vi "Interpolate_Calib_Coeff.vi"(5 "Analysis Info cluster":T1={"Colour"=0, "Inst type"=enum."Pitot-static tube", "Inst name"="Manometer voltage", "Symbol"="U", "Code name"="", "Extra Info"="U", "Inst Array"=enum."PWA", "Extra Titles"=[], "Extra Values"=[], "U"=0.0, "u^2"=0.0, "u^3"=0.0, "u^4"=0.0, "Skew_u"=0.0, "Kurt_u"=0.0, "Sd Error in Mean"=0.0, "% u'/U"=0.0, "X"=0.0, "Y"=0.0, "Z"=0.0, "Timescale integral to 25%"=0.0, "Sd Error in Variance"=0.0, "Calib File"=path "", "Calib Constants"=[], "Output Position"=FALSE, "Full Stats"=FALSE, "Av Sampling Rate"=0.0, "Av No of Samples"=0.0, "Total Meas Time (s)"=0.0, "ADAM Ch Name"="", "Max value"=0.0, "Min value"=0.0} {"Sd Error in Variance" format="%.2f"; "Skew_u" format="%.2f"; "% u'/U" format="%.2f"; "Sd Error in Mean" format="%.2f"; "Kurt_u" format="%.2f"; "u^4" format="%.2f"; "u^3" format="%.2f"; "U" format="%.2f"; "u^2" format="%.2f"}, 7 "Take New Data?":bool) -> (0 "Calib Coeff":dbl[](array[numeric]), 1 "Calib Type Name":string, 2 "Calib file string":string, 3 "Read file":bool, 4 "Analysis Info cluster  Out":T1={"Colour"=0, "Inst type"=enum."Pitot-static tube", "Inst name"="Manometer voltage", "Symbol"="U", "Code name"="", "Extra Info"="U", "Inst Array"=enum."PWA", "Extra Titles"=[], "Extra Values"=[], "U"=0.0, "u^2"=0.0, "u^3"=0.0, "u^4"=0.0, "Skew_u"=0.0, "Kurt_u"=0.0, "Sd Error in Mean"=0.0, "% u'/U"=0.0, "X"=0.0, "Y"=0.0, "Z"=0.0, "Timescale integral to 25%"=0.0, "Sd Error in Variance"=0.0, "Calib File"=path "", "Calib Constants"=[], "Output Position"=FALSE, "Full Stats"=FALSE, "Av Sampling Rate"=0.0, "Av No of Samples"=0.0, "Total Meas Time (s)"=0.0, "ADAM Ch Name"="", "Max value"=0.0, "Min value"=0.0} {"Sd Error in Variance" format="%.2f"; "Skew_u" format="%.2f"; "% u'/U" format="%.2f"; "Sd Error in Mean" format="%.2f"; "Kurt_u" format="%.2f"; "u^4" format="%.2f"; "u^3" format="%.2f"; "U" format="%.2f"; "u^2" format="%.2f"})   [LabVIEW 2015]
uses:
  Controls/Analysis_info_cluster.ctl
  Controls/Inst_type.ctl
  Controls/Instrument_Array.ctl
  XW calib map/Map method.ctl
  Globals/Meas_global.vi
  XW calib map/XW_Map_Global.vi
  Globals/Plug_in_data_global.vi
  Globals/Dynamic_call_global.ph.vi
  <vilib>/Analysis/NI_AALPro.lvlib
panel:
  out "Volts":dbl
  out "Time":dbl format="%#.0f"
  out "Earlier raw data file":string
  in  "TAKE NEW DATA XW Map method":T4=enum."Const. Psi_eff (std.)"
  in  "Domain padding factor":dbl=1.01
  in  "cap indicial sum to n":bool=TRUE
  in  "surface order (n)":i32=5
  in  "Apply calibration corrections":bool=TRUE
  in  "POST PROC. XW Map method":T4=enum."Psi_eff, k = f(Umagn.)"
  in  "variable n":bool=TRUE
  in  "wire diameter (mu.m)":dbl=5.0
  out "Header info":string[][](array[string])
  # "For polysurface method only:"
  # "For trimesh method only"
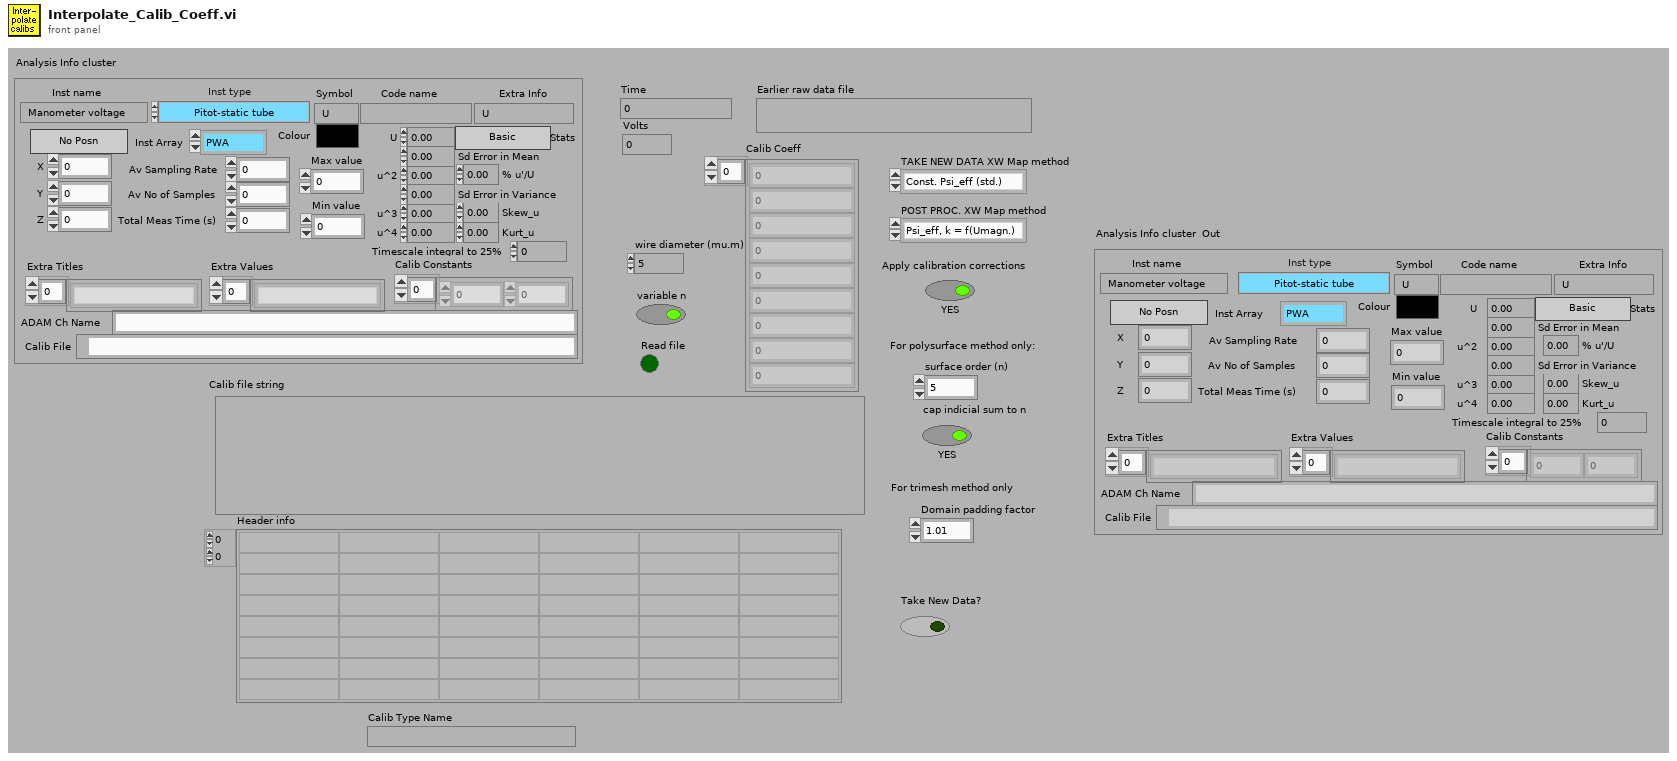
[diagram p1: front panel]
types:
  T1 = typedef "Analysis_info_cluster.ctl" = cluster{"Colour":u32, "Inst type":T2, "Inst name":string, "Symbol":string, "Code name":string, "Extra Info":string, "Inst Array":T3, "Extra Titles":string[], "Extra Values":string[], "U":dbl, "u^2":dbl, "u^3":dbl, "u^4":dbl, "Skew_u":dbl, "Kurt_u":dbl, "Sd Error in Mean":dbl, "% u'/U":dbl, "X":dbl, "Y":dbl, "Z":dbl, "Timescale integral to 25%":dbl, "Sd Error in Variance":dbl, "Calib File":path, "Calib Constants":dbl[], "Output Position":bool, "Full Stats":bool, "Av Sampling Rate":dbl, "Av No of Samples":dbl, "Total Meas Time (s)":dbl, "ADAM Ch Name":string, "Max value":dbl, "Min value":dbl}
  T2 = typedef "Inst_type.ctl" = enum16{"Propeller anemometer", "Raw voltage", "Pressure Transducer", "Pitot-static tube", "Preston tube", "Hot wire", "Cross wire 1", "Cross wire 2", "Generic Linear", "Generic Polynomial", "Generic BackPoly", "Fast FID", "Thermocouple", "Cold wire", "Pulsed Wire", "LDA Vel", "LDA Tran time", "LDA Arr time", "Microphone"}
  T3 = typedef "Instrument_Array.ctl" = enum16{"PWA", "LDA", "Analogue"}
  T4 = typedef "Map method.ctl" = enum16{"Triangle mesh", "Polynomial surface", "Const. Psi_eff (std.)", "Psi_eff = f(Umagn.)", "Psi_eff, k = f(Umagn.)"}
  T5 = cluster{"1st Calib time":dbl, "2nd Calib time":dbl, "Meas start time":dbl, "Meas end time":dbl, "Fraction":dbl}
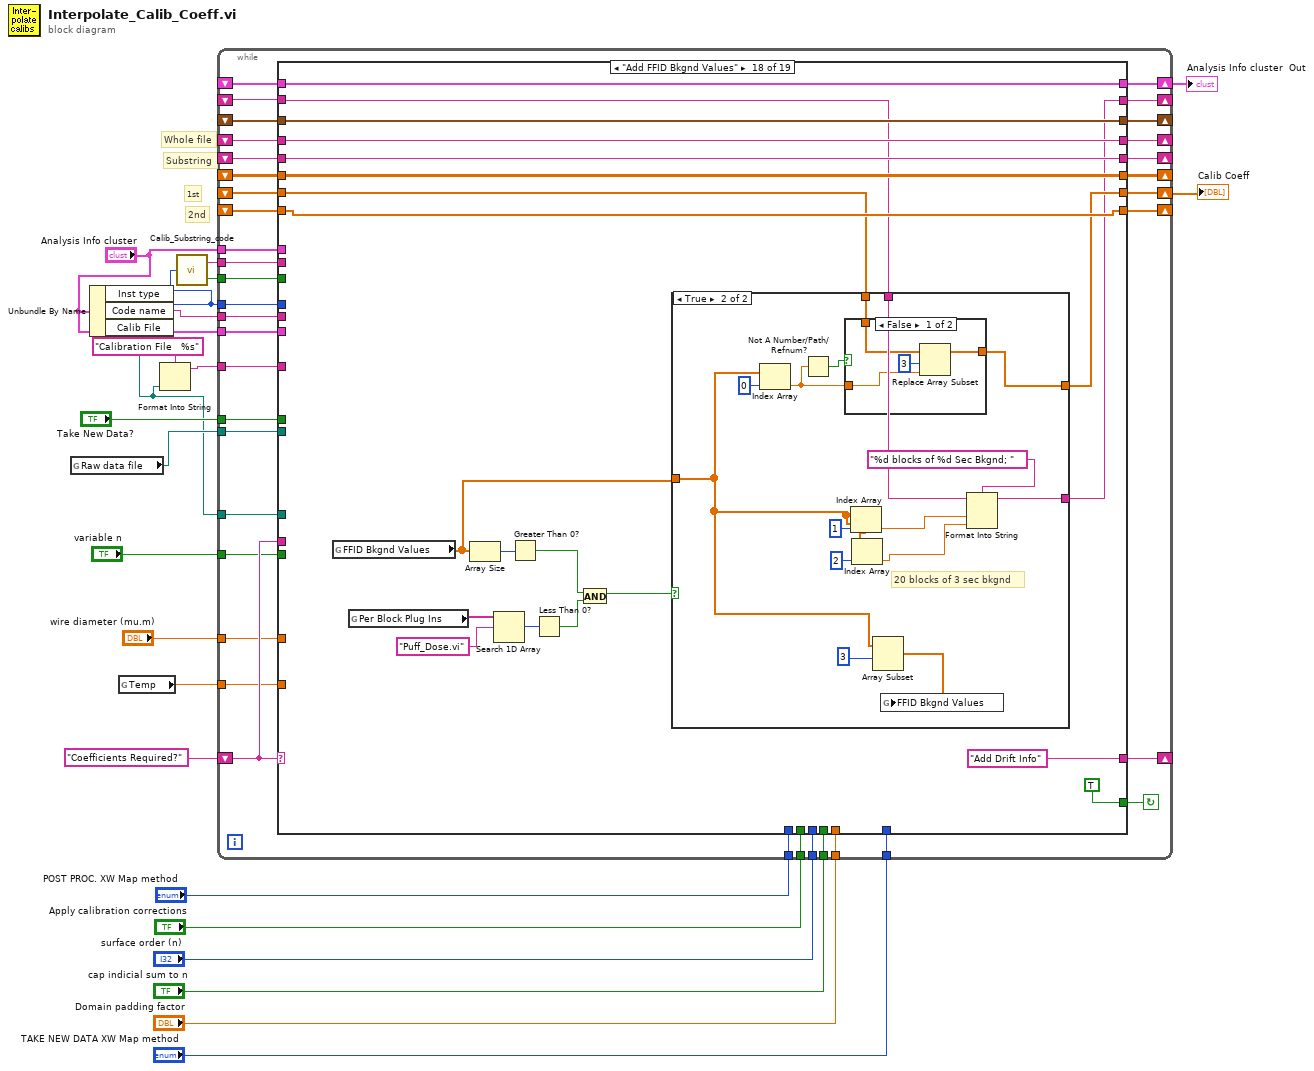
[diagram p0: block diagram]
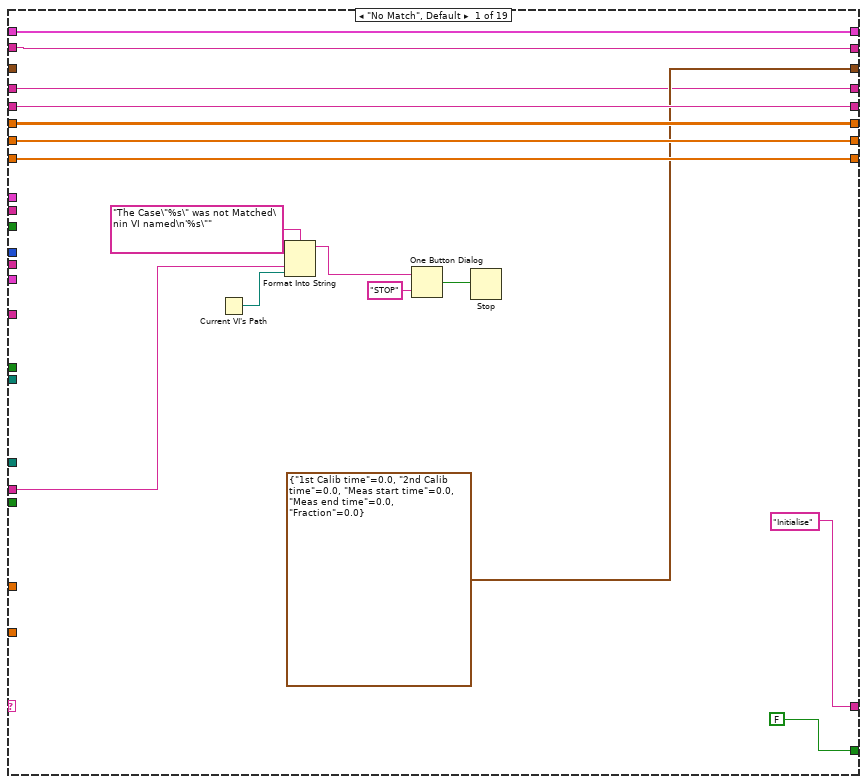
[diagram p2: hidden frame]
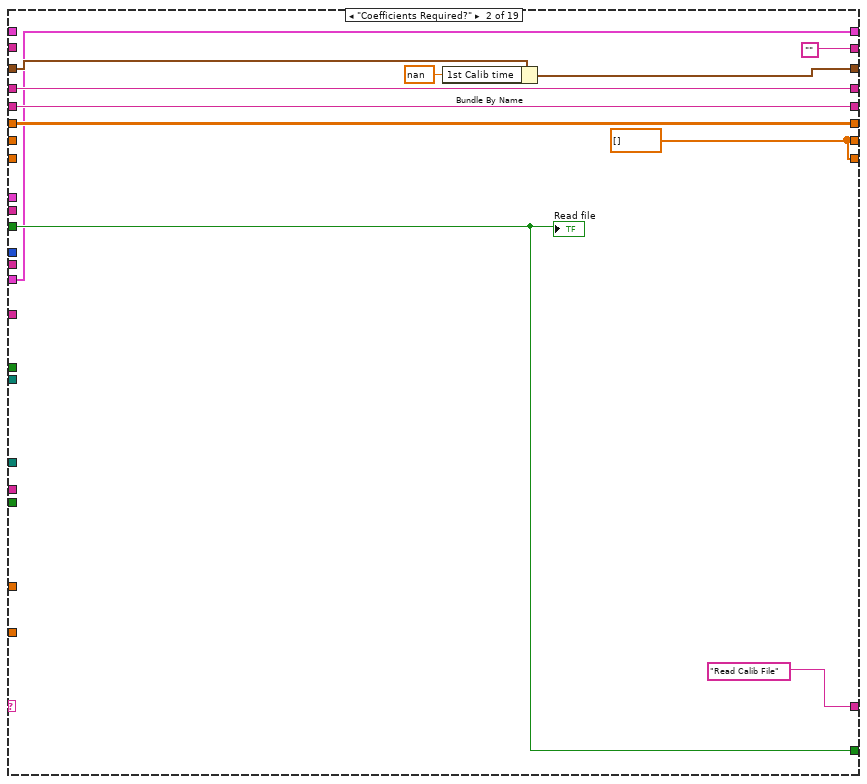
[diagram p3: hidden frame]
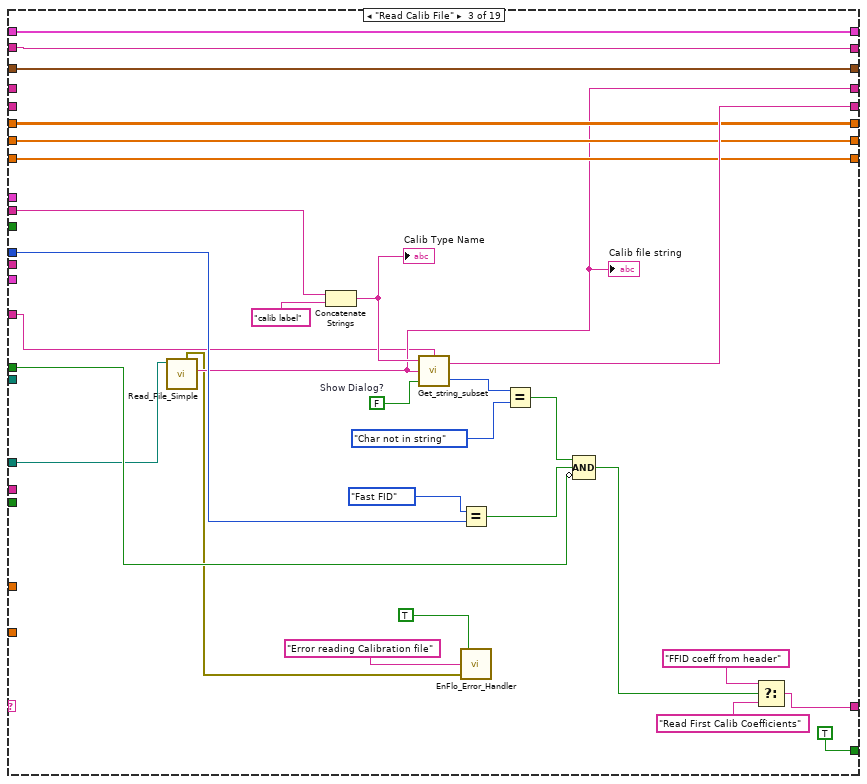
[diagram p4: hidden frame]
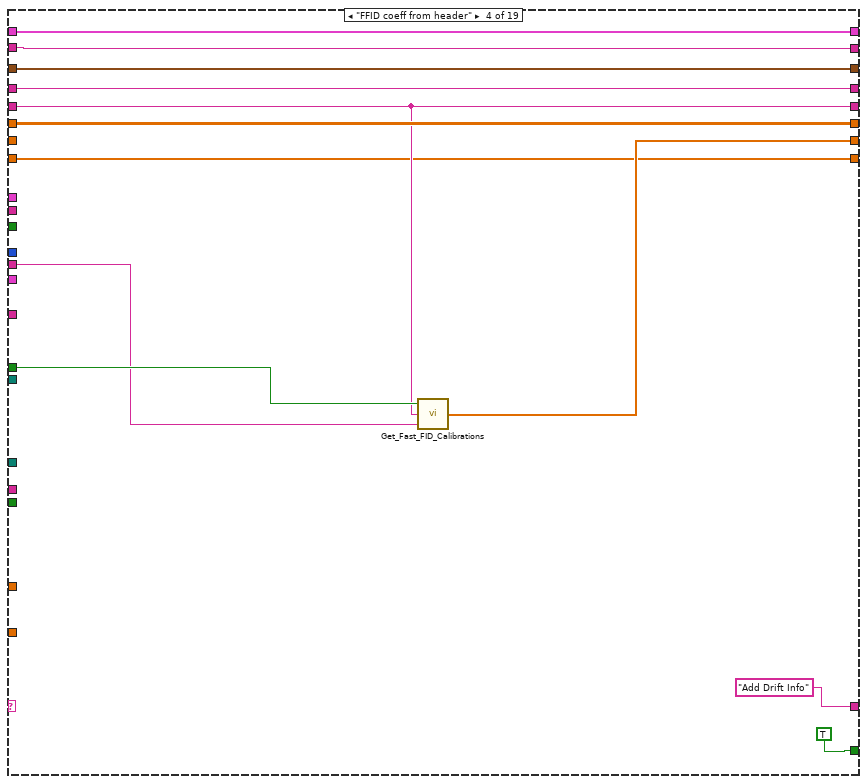
[diagram p5: hidden frame]
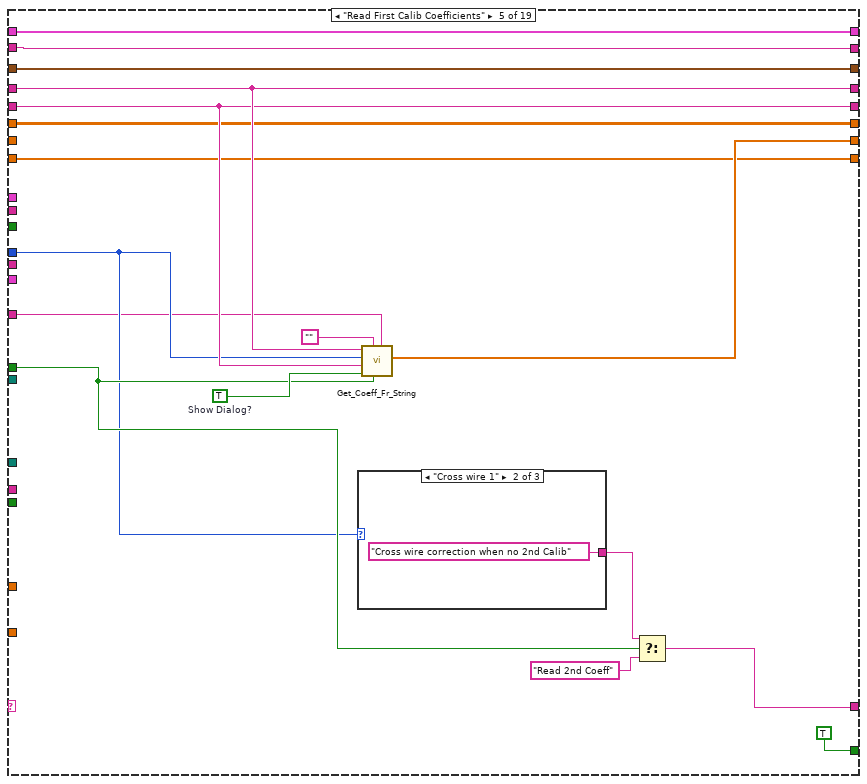
[diagram p6: hidden frame]
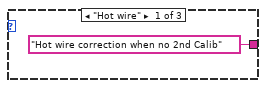
[diagram p7: hidden frame]
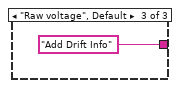
[diagram p8: hidden frame]
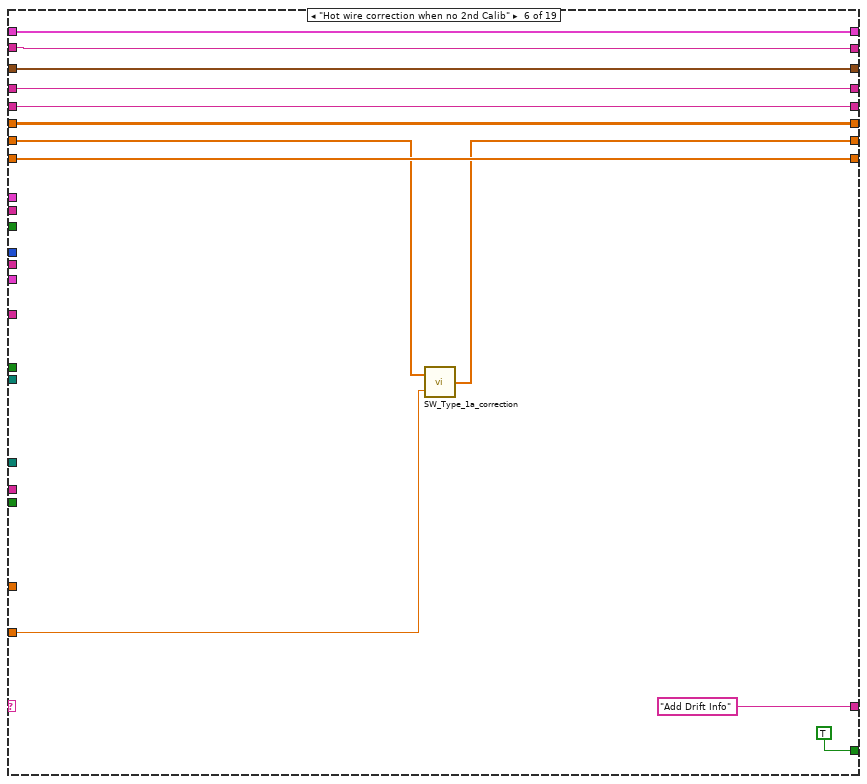
[diagram p9: hidden frame]
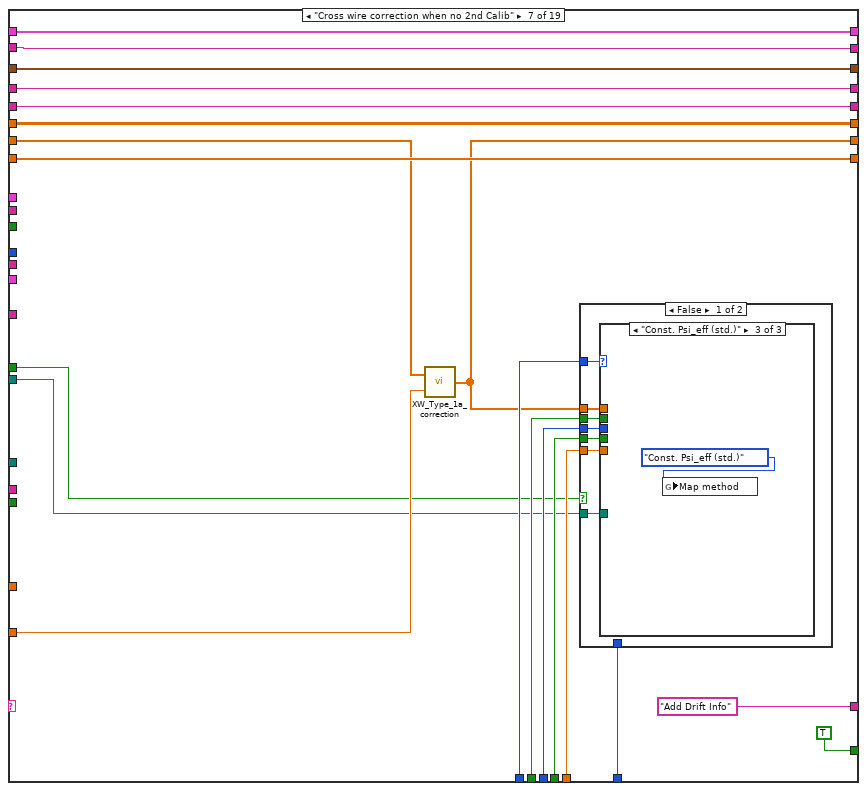
[diagram p10: hidden frame]
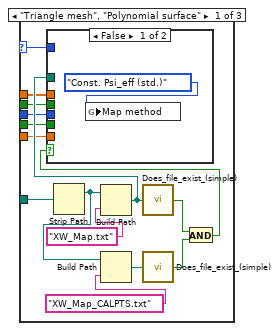
[diagram p11: hidden frame]
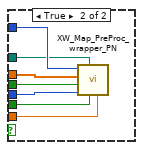
[diagram p12: hidden frame]
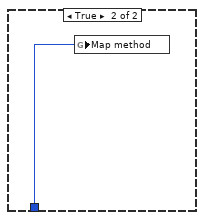
[diagram p14: hidden frame]
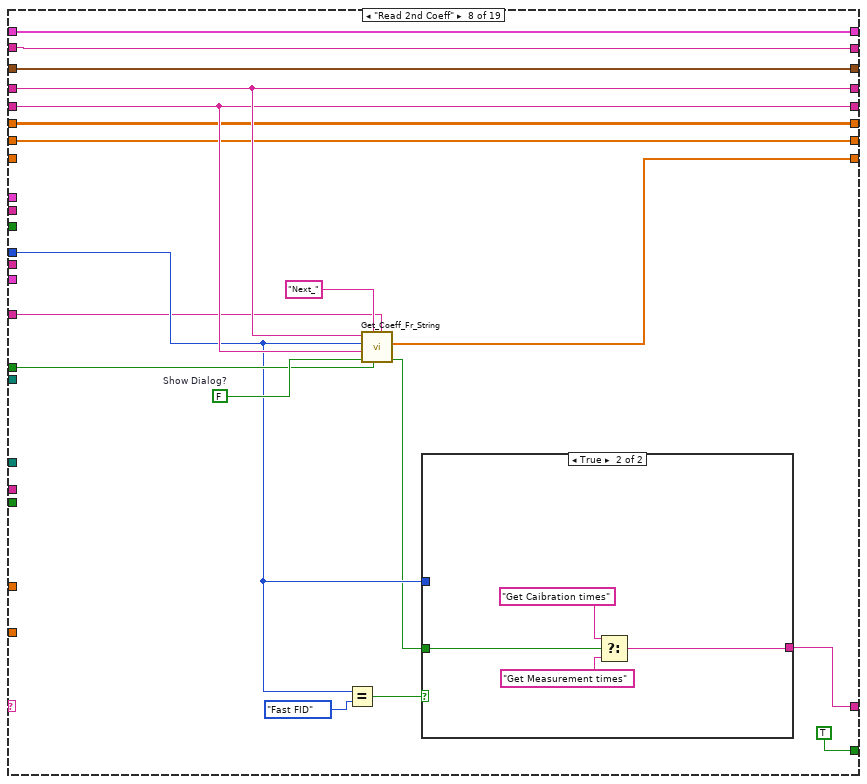
[diagram p15: hidden frame]
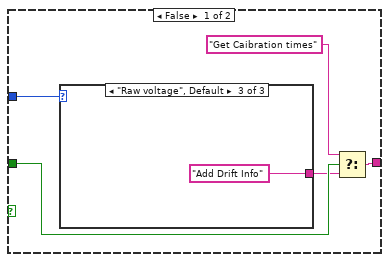
[diagram p16: hidden frame]
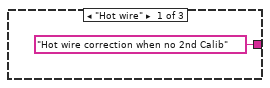
[diagram p17: hidden frame]
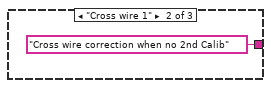
[diagram p18: hidden frame]
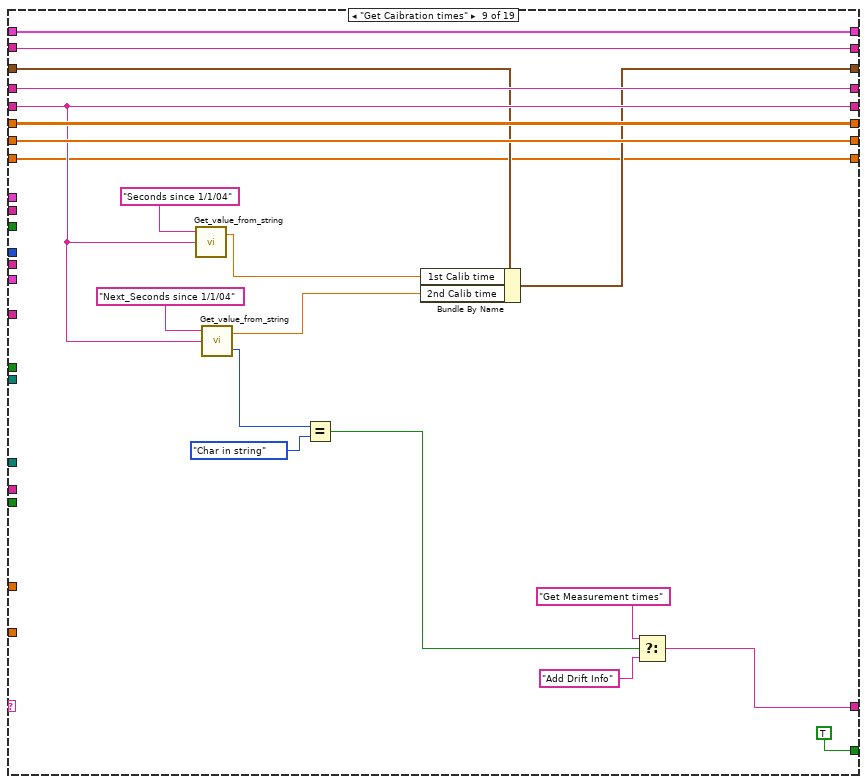
[diagram p19: hidden frame]
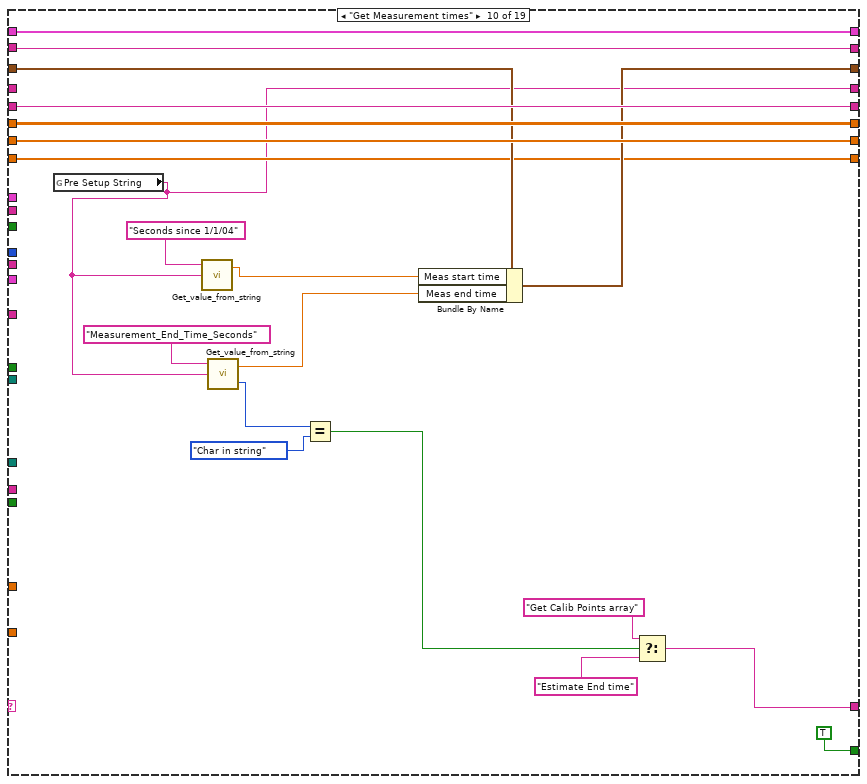
[diagram p20: hidden frame]
diagram:
  # "Substring"
  # "2nd"
  # "Whole file"
  # "1st"
  n1 = global read "Meas_global.vi" "Raw data file"() -> (w15:path)
  n2 = Unbundle By Name("Analysis Info cluster") -> ("Inst type"=w18:T2, "Code name"=w19:string, "Calib File"=w1:path)
  n3 = global read "Meas_global.vi" "Temp"() -> (w14:dbl)
  n4 = Format Into String(format string="Calibration File   %s", w1) -> (resulting string=w2:string)  [unwired: 2 in, 1 out]
  n5 = call "Calib_Substring_code.vi"("Inst type"=w18) -> ("Substring Type"=w16:string, "Read file"=w17:bool)
  n6 = while {
    tunnel: w1 -> [w51]
    shift-left: _ -> [w52]
    shift-right: [w53] -> _
    shift-left: _ -> [w54]
    shift-right: [w56] -> w21
    tunnel: w18 -> [w58]
    shift-left: _ -> [w55]
    shift-right: [w57] -> _
    shift-left: "Coefficients Required?" -> [w59]
    shift-right: [w24] -> _
    tunnel: "Take New Data?" -> [w50]
    tunnel: w19 -> [w49]
    shift-right: [w48] -> _
    shift-left: _ -> [w47]
    shift-right: [w46] -> _
    shift-left: _ -> [w45]
    shift-right: [w44] -> _
    shift-left: _ -> [w43]
    tunnel: w17 -> [w42]
    tunnel: w16 -> [w41]
    tunnel: w15 -> [w40]
    shift-right: [w39] -> _
    shift-left: _ -> [w38]
    tunnel: w14 -> [w37]
    tunnel: "wire diameter (mu.m)" -> [w36]
    tunnel: "variable n" -> [w35]
    tunnel: "POST PROC. XW Map method" -> [w34]
    tunnel: "Apply calibration corrections" -> [w33]
    tunnel: "surface order (n)" -> [w32]
    tunnel: "cap indicial sum to n" -> [w31]
    tunnel: "Domain padding factor" -> [w30]
    tunnel: "TAKE NEW DATA XW Map method" -> [w29]
    tunnel: "Analysis Info cluster" -> [w28]
    shift-right: [w26] -> w5
    shift-left: _ -> [w27]
    tunnel: "Analysis Info cluster" -> [w25]
    tunnel: w2 -> [w23]
    stop <- w60 continue-if-true
    n7 = case shown="\"Add FFID Bkgnd Values\"" w59 {
      tunnel: [FALSE w82 TRUE ("Read file") TRUE TRUE ("Read file") TRUE ("Read file") TRUE ("Read file") TRUE ("Read file") TRUE ("Read file") TRUE ("Read file") TRUE ("Read file") TRUE ("Read file") TRUE ("Read file") TRUE ("Read file") TRUE ("Read file") w501 w911 TRUE ("Read file") FALSE ("Read file")] -> w60
      tunnel: ["Initialise" "Read Calib File" w102 "Add Drift Info" w132 "Add Drift Info" "Add Drift Info" w224 w259 w280 w294 w329 "Bkgnd info from header" ("f") "Add Drift Info" ("f") "Add Drift Info" ("f") w502 w912 "Add Drift Info" "End"] -> w24
      tunnel: w59 -> [w71 _ _ _ _ _ _ _ _ _ _ _ _ _ _ _ _ _ _]
      tunnel: w58 -> [_ _ w109 _ w134 _ _ w216 _ _ _ w315 _ _ _ _ _ _ _]
      tunnel: [w68 w86 w115 w124 w142 w159 w179 w228 w253 w274 w308 w333 w375 w408 w454 w509 w919 w1008 w1042] -> w57
      tunnel: [w67 w84 w99 w122 w144 w151 w162 w222 w258 w279 w309 w332 w348 w407 w414 w505 w915 w1000 w1036] -> w56
      tunnel: w55 -> [w68 w86 _ w124 w142 w159 w179 w228 w253 w274 w308 w333 w375 w408 w454 w510 w920 w1008 w1042]
      tunnel: w54 -> [w67 _ w99 _ _ w152 w170 w222 w258 w279 w309 w332 w347 w394 w438 w506 w916 w1001 w1051]
      tunnel: [w66 w85 w114 w128 w141 w158 w178 w227 w261 w282 w311 w331 w364 w390 w428 w508 w918 w1004 w1060] -> w53
      tunnel: w52 -> [w66 w85 w114 w128 w141 w158 w178 w227 w261 w282 w311 _ w364 w390 w428 w507 w917 w1004 w1060]
      tunnel: w51 -> [_ _ w89 _ _ _ _ _ _ _ _ _ _ _ _ _ _ _ _]
      tunnel: w50 -> [_ _ w105 w125 w138 _ w165 w225 _ _ _ _ _ _ w416 _ _ _ w1034]
      tunnel: w49 -> [_ _ _ w123 _ _ _ _ _ _ _ _ _ _ _ w513 w923 _ _]
      tunnel: [w65 w84 w98 w121 w140 w157 w177 w221 w245 w266 w306 w316 w368 w393 w439 w504 w914 w1007 w1059] -> w48
      tunnel: w47 -> [w65 _ w98 w121 w140 w157 w177 _ w245 w266 w306 w316 w368 w393 w439 w503 w913 w1007 w1059]
      tunnel: [w63 w83 w97 w119 w143 w160 w180 w229 w262 w265 w305 w328 w365 w404 w451 w511 w921 w1005 w1061] -> w46
      tunnel: w45 -> [w63 w83 _ w119 w143 w160 w180 w229 w262 _ w305 w328 w365 w404 w451 w514 w924 w1005 w1061]
      tunnel: [T5 {"1st Calib time"=0.0, "2nd Calib time"=0.0, "Meas start time"=0.0, "Meas end time"=0.0, "Fraction"=0.0} w80 w96 w120 w137 w155 w175 w220 w249 w270 w307 w317 w366 w405 w452 w500 w910 w1006 w1039] -> w44
      tunnel: w43 -> [_ w81 w96 w120 w137 w155 w175 w220 w252 w273 w304 w319 w366 w405 w452 w512 w922 w1006 w1039]
      tunnel: w42 -> [_ w82 _ _ _ _ _ _ _ _ _ _ _ _ _ _ _ _ _]
      tunnel: w41 -> [_ _ w95 _ _ _ _ _ _ _ _ _ _ _ _ _ _ _ _]
      tunnel: w40 -> [_ _ _ _ _ _ w164 _ _ _ w292 _ _ _ w417 w496 _ _ w1035]
      tunnel: [w62 "" w94 w118 w135 w154 w174 w217 w244 w264 w293 w313 w355 w396 w443 w499 w908 w998 w1038] -> w39
      tunnel: w38 -> [w62 _ w94 w118 w135 w154 w174 w217 w244 w264 w293 w313 w357 w398 w445 w498 w909 w999 w1038]
      tunnel: w37 -> [_ _ _ _ _ w150 w172 _ _ _ _ _ _ w385 w419 _ _ _ _]
      tunnel: w36 -> [_ _ _ _ _ _ _ _ _ _ _ _ _ w383 w418 _ _ _ _]
      tunnel: w35 -> [_ _ _ _ _ _ _ _ _ _ _ _ _ w384 w420 _ _ _ _]
      tunnel: w34 -> [_ _ _ _ _ _ w171 _ _ _ _ _ _ _ w415 _ _ _ w1033]
      tunnel: w33 -> [_ _ _ _ _ _ w169 _ _ _ _ _ _ _ w413 _ _ _ _]
      tunnel: w32 -> [_ _ _ _ _ _ w168 _ _ _ _ _ _ _ w412 _ _ _ _]
      tunnel: w31 -> [_ _ _ _ _ _ w167 _ _ _ _ _ _ _ w411 _ _ _ _]
      tunnel: w30 -> [_ _ _ _ _ _ w166 _ _ _ _ _ _ _ w410 _ _ _ _]
      tunnel: w29 -> [_ _ _ _ _ _ w163 _ _ _ _ _ _ _ _ _ _ _ _]
      tunnel: w28 -> [_ w77 _ _ _ _ _ _ _ _ _ _ _ _ _ _ _ _ w1032]
      tunnel: w27 -> [w61 _ w90 w117 w131 w149 w161 w214 w243 w263 w289 w312 w354 w382 w409 w497 w907 w997 _]
      tunnel: [w61 w77 w90 w117 w131 w149 w161 w214 w243 w263 w289 w312 w354 w382 w409 w497 w907 w997 w1031] -> w26
      tunnel: w25 -> [_ _ _ _ _ _ _ _ _ _ _ _ _ _ _ _ _ _ _]
      tunnel: w23 -> [_ _ w88 _ w130 _ _ w213 _ _ _ _ _ _ _ _ _ _ _]
      frame "No Match", Default {
        n8 = Current VI's Path() -> (path=w70:path)
        n9 = Format Into String(format string="The Case\"%s\" was not Matched\nin VI named\n'%s\"" ("Format String"), w71, w70) -> (resulting string=w74:string)  [unwired: 2 in, 1 out]
        n10 = One Button Dialog(message=w74, button name ("OK")="STOP") -> (true=w72:bool)
        n11 = Stop(stop? (T)=w72) -> ()
      }
      frame "Coefficients Required?" {
        w84 = dbl[] [] ("Calib Coeff")
        n12 = Bundle By Name(cluster=w81, "1st Calib time"=nan) -> (w80:T5)
        "Read file" <- w82
      }
      frame "Read Calib File" {
        w110 = FALSE  # Show Dialog?
        n13 = call "Read_File_Simple.vi"("Filename"=w89) -> ("error out"=w93:errorcluster, "string"=w97:string)  [unwired: 2 in, 6 out]
        "Calib file string" <- w97
        n14 = Concatenate Strings(w95, "calib label") -> (w113:string)
        "Calib Type Name" <- w113
        n15 = call "Get_string_subset.vi"("String Name"=w88, "Show Dialog?"=w110, "String to split"=w97, "File Label"=w113) -> ("Status"=w112:enum16{"Char in string", "Char not in string"}, "Output string"=w115:string)
        n16 = Equal?(x=Inst_type."Fast FID" ("Inst type"), y=w109) -> (x = y?=w106:bool)
        n17 = call "EnFlo_Error_Handler.vi"("error in (no error)"=w93, "Error Type"="Error reading Calibration file", "Dialog Box (T)"=TRUE) -> ()  [unwired: 3 out]
        n18 = Equal?(x=w112, y=enum16{"Char in string", "Char not in string"}."Char not in string" ("Status")) -> (x = y?=w107:bool)
        n19 = Compound Arithmetic op=AND(w107, w106, invert w105) -> (w103:bool)
        n20 = Select(t="FFID coeff from header", s=w103, f="Read First Calib Coefficients") -> (s? t:f=w102:string)
      }
      frame "FFID coeff from header" {
        n21 = call "Get_Fast_FID_Calibrations.vi"("Code Name"=w123, "Calib File String"=w124, "Take New Data"=w125) -> ("Calib Constants"=w122:dbl[])
      }
      frame "Read First Calib Coefficients" {
        w145 = TRUE  # Show Dialog?
        n22 = case shown="\"Cross wire 1\"" w134 {
          tunnel: ["Hot wire correction when no 2nd Calib" "Cross wire correction when no 2nd Calib" "Add Drift Info"] -> w133
          frame "Hot wire" {
          }
          frame "Cross wire 1" {
          }
          frame "Raw voltage", Default {
          }
        }
        n23 = call "Get_Coeff_Fr_String.vi"("String Name"=w130, "Take New Data?"=w138, "Prefix"="", "Show Dialog?"=w145, "Sub String"=w142, "Inst type"=w134, "Whole String"=w143) -> ("Calib Constants"=w144:dbl[])  [unwired: 2 in, 1 out]
        n24 = Select(t=w133, s=w138, f="Read 2nd Coeff") -> (s? t:f=w132:string)
      }
      frame "Hot wire correction when no 2nd Calib" {
        n25 = call "SW_Type_1a_correction.vi"("Tmeas (degC)"=w150, "Calib consts."=w152) -> ("Corrected calib consts."=w151:dbl[])
      }
      frame "Cross wire correction when no 2nd Calib" {
        n26 = call "XW_Type_1a_correction.vi"("Tmeas (degC)"=w172, "Calib consts."=w170) -> ("Corrected calib consts."=w162:dbl[])
        n27 = case shown="False" w165 {
          tunnel: w164 -> [w187 _]
          tunnel: w171 -> [w181 _]
          tunnel: w162 -> [w186 _]
          tunnel: w169 -> [w185 _]
          tunnel: w168 -> [w184 _]
          tunnel: w167 -> [w183 _]
          tunnel: w166 -> [w182 _]
          tunnel: w163 -> [_ w212]
          frame False {
            n28 = case shown="\"Const. Psi_eff (std.)\"" w181 {
              selector: w181 -> [w194 _ _]
              tunnel: w187 -> [w202 _ _]
              tunnel: w186 -> [w199 _ _]
              tunnel: w185 -> [w198 _ _]
              tunnel: w184 -> [w197 _ _]
              tunnel: w183 -> [w196 _ _]
              tunnel: w182 -> [w195 _ _]
              frame "Triangle mesh", "Polynomial surface" {
                n29 = Strip Path(path=w202) -> (stripped path=w191:path)  [unwired: 1 out]
                n30 = Build Path(base path=w191, name or relative path="XW_Map.txt") -> (appended path=w200:path)
                n31 = Build Path(base path=w191, name or relative path="XW_Map_CALPTS.txt") -> (appended path=w193:path)
                n32 = call "Does_file_exist_(simple).vi"("Pathname"=w200) -> ("exists?"=w189:bool)
                n33 = call "Does_file_exist_(simple).vi"("Pathname"=w193) -> ("exists?"=w190:bool)
                n34 = And(x=w189, y=w190) -> (x .and. y?=w188:bool)
                n35 = case shown="False" w188 {
                  tunnel: w200 -> [_ w209]
                  tunnel: w194 -> [_ w210]
                  tunnel: w199 -> [_ w208]
                  tunnel: w198 -> [_ w207]
                  tunnel: w197 -> [_ w206]
                  tunnel: w196 -> [_ w205]
                  tunnel: w195 -> [_ w204]
                  frame False {
                    n36 = global write "XW_Map_Global.vi" "Map method"(Map_method."Const. Psi_eff (std.)" ("Map method")) -> ()
                  }
                  frame True {
                    n37 = call "XW_Map_PreProc_wrapper_PN.vi"("Domain padding factor"=w204, "cap indicial sum to n"=w205, "XW_Calib_Map file path"=w209, "surface order (n)"=w206, "Apply calibration corrections"=w207, "Calib const"=w208, "Map method"=w210) -> ()  [unwired: 5 out]
                  }
                }
              }
              frame "Psi_eff = f(Umagn.)", "Psi_eff, k = f(Umagn.)" {
              }
              frame "Const. Psi_eff (std.)" {
                n38 = global write "XW_Map_Global.vi" "Map method"(Map_method."Const. Psi_eff (std.)" ("Map method")) -> ()
              }
            }
          }
          frame True {
            n39 = global write "XW_Map_Global.vi" "Map method"(w212) -> ()
          }
        }
      }
      frame "Read 2nd Coeff" {
        w230 = FALSE  # Show Dialog?
        n40 = Equal?(x=w216, y=Inst_type."Fast FID" ("Inst type")) -> (x = y?=w218:bool)
        n41 = call "Get_Coeff_Fr_String.vi"("String Name"=w213, "Take New Data?"=w225, "Prefix"="Next_", "Show Dialog?"=w230, "Sub String"=w228, "Inst type"=w216, "Whole String"=w229) -> ("Coefficients Found?"=w215:bool, "Calib Constants"=w221:dbl[])  [unwired: 2 in]
        n42 = case shown="True" w218 {
          tunnel: [w231 w242] -> w224
          tunnel: w215 -> [w233 w239]
          tunnel: w216 -> [w235 _]
          frame False {
            n43 = case shown="\"Raw voltage\", Default" w235 {
              tunnel: ["Hot wire correction when no 2nd Calib" "Cross wire correction when no 2nd Calib" "Add Drift Info"] -> w232
              frame "Hot wire" {
              }
              frame "Cross wire 1" {
              }
              frame "Raw voltage", Default {
              }
            }
            n44 = Select(t="Get Caibration times", s=w233, f=w232) -> (s? t:f=w231:string)
          }
          frame True {
            n45 = Select(t="Get Caibration times", s=w239, f="Get Measurement times") -> (s? t:f=w242:string)
          }
        }
      }
      frame "Get Caibration times" {
        n46 = call "Get_value_from_string.vi"("Input string"=w253, "Variable name"="Seconds since 1/1/04") -> ("Value"=w251:dbl)  [unwired: 1 in, 1 out]
        n47 = call "Get_value_from_string.vi"("Input string"=w253, "Variable name"="Next_Seconds since 1/1/04") -> ("Status"=w248:enum16{"Char in string", "Char not in string"}, "Value"=w250:dbl)  [unwired: 1 in]
        n48 = Equal?(x=w248, y=enum16{"Char in string", "Char not in string"}."Char in string" ("Status")) -> (x = y?=w246:bool)
        n49 = Bundle By Name(cluster=w252, "1st Calib time"=w251, "2nd Calib time"=w250) -> (w249:T5)
        n50 = Select(t="Get Measurement times", s=w246, f="Add Drift Info") -> (s? t:f=w259:string)
      }
      frame "Get Measurement times" {
        n51 = global read "Meas_global.vi" "Pre Setup String"() -> (w265:string)
        n52 = call "Get_value_from_string.vi"("Input string"=w265, "Variable name"="Seconds since 1/1/04") -> ("Value"=w272:dbl)  [unwired: 1 in, 1 out]
        n53 = call "Get_value_from_string.vi"("Input string"=w265, "Variable name"="Measurement_End_Time_Seconds") -> ("Status"=w269:enum16{"Char in string", "Char not in string"}, "Value"=w271:dbl)  [unwired: 1 in]
        n54 = Equal?(x=w269, y=enum16{"Char in string", "Char not in string"}."Char in string" ("Status")) -> (x = y?=w267:bool)
        n55 = Bundle By Name(cluster=w273, "Meas start time"=w272, "Meas end time"=w271) -> (w270:T5)
        n56 = Select(t="Get Calib Points array", s=w267, f="Estimate End time") -> (s? t:f=w280:string)
      }
      frame "Estimate End time" {
        n57 = Unbundle By Name(w304) -> ("Meas start time"=w303:dbl)
        n58 = call "Read_RD_Ch_header.vi"("Raw data file"=w292) -> ("Ch Name Out"=w291:string[], "Ch Values"=w290:string[])  [unwired: 2 out]
        n59 = Search 1D Array(1D array=w291, element="Flow:Measurement:Time") -> (index of element=w300:i32)  [unwired: 1 out]
        n60 = Index Array(array=w290, index=w300) -> (element=w285:string)
        n61 = Search and Replace String(input string=w285, search string=",", replace string="." ("replace string (\"\")")) -> (result string=w286:string)  [unwired: 5 in, 3 out]
        n62 = Fract/Exp String To Number(string=w286, default (0 dbl)=nan ("default (0 DBL)")) -> (number=w283:dbl)  [unwired: 3 out]
        n63 = Not A Number/Path/Refnum?(number/path/refnum=w283) -> (NaN/Path/Refnum?=w297:bool)
        n64 = Multiply(x=w283, y=60.0) -> (x*y=w298:dbl)
        n65 = Add(x=w303, y=w298) -> (x+y=w302:dbl)
        n66 = Bundle By Name(cluster=w304, "Meas end time"=w302) -> (w307:T5)
        n67 = Select(t="Add Drift Info", s=w297, f="Get Calib Points array") -> (s? t:f=w294:string)
      }
      frame "Get Calib Points array" {
        w335 = FALSE  # Show Dialog?
        # "Fraction = (Av_Meas_Time - Calib1_time)  /  (Calib2_time - Calib1_time)"
        n68 = Unbundle By Name(w319) -> ("Meas start time"=w324:dbl, "Meas end time"=w323:dbl, "2nd Calib time"=w325:dbl, "1st Calib time"=w314:dbl)
        n69 = Add(x=w324, y=w323) -> (x+y=w327:dbl)
        n70 = call "2D_array_from_string.vi"("Show Dialog?"=w335, "Input string"=w333, "Array title"="Calib points label") -> ("2D data array"=w331:dbl[][])  [unwired: 1 in]
        n71 = Divide(x=w327, y=2.0) -> (x/y=w322:dbl)
        n72 = Subtract(x=w325, y=w314) -> (x-y=w320:dbl)
        n73 = Subtract(x=w322, y=w314) -> (x-y=w321:dbl)
        n74 = Divide(x=w321, y=w320) -> (x/y=w318:dbl)
        n75 = case shown="\"Propeller anemometer\", Default" w315 {
          tunnel: ["Add Drift Info" "Single Hot wire" "Cross wire" w340] -> w329
          tunnel: w314 -> [_ _ _ w343]
          frame "Propeller anemometer", Default {
          }
          frame "Hot wire" {
          }
          frame "Cross wire 1" {
          }
          frame "Fast FID" {
            n76 = Not A Number/Path/Refnum?(number/path/refnum=w343) -> (NaN/Path/Refnum?=w342:bool)
            n77 = Select(t="Bkgnd info from header", s=w342, f="Fast FID") -> (s? t:f=w340:string)
          }
        }
        n78 = Bundle By Name(cluster=w319, "Fraction"=w318) -> (w317:T5)
      }
      frame "Fast FID" {
        # "Concentrations"
        # "Voltage"
        # "End"
        # "Start"
        # "(End-Start)*Fraction + Start"
        n79 = Index Array(array=w364, index (col)=1) -> (element=w371:dbl[])  [unwired: 1 in]
        n80 = call "2nd_order_Poly_convert.vi"("Calib constants"=w368, "Voltage"=w371) -> ("Eng Values"=w372:dbl[])  [unwired: 4 out]
        n81 = call "2nd_order_Poly_convert.vi"("Calib constants"=w347, "Voltage"=w371) -> ("Eng Values"=w373:dbl[])  [unwired: 4 out]
        n82 = Unbundle By Name(w366) -> ("Fraction"=w361:dbl)
        n83 = In Range and Coerce(upper limit=1.0, x=w361, lower limit=0.0) -> (coerced(x)=w358:dbl)  [unwired: 1 out]
        n84 = for {
          tunnel: w373 -> [w377] mode=indexing
          tunnel: w372 -> [w381] mode=indexing
          tunnel: w358 -> [w379]
          tunnel: [w376] -> w370 mode=indexing
          n85 = Subtract(x=w381, y=w377) -> (x-y=w380:dbl)
          n86 = Multiply(x=w379, y=w380) -> (x*y=w378:dbl)
          n87 = Add(x=w377, y=w378) -> (x+y=w376:dbl)
        }
        n88 = Index Array(array=w347, index=5) -> (element=w345:dbl)
        n89 = Format Into String(format string="Calib Fraction %.4f; ", initial string=w357, w358) -> (resulting string=w355:string)  [unwired: 1 in, 1 out]
        n90 = Build Array(w345) -> (w344:dbl[])
        n91 = call <vilib>:"General Polynomial Fit.vi"("Y"=w370, "polynomial order"=2, "X"=w371) -> ("Polynomial Coefficients"=w350:dbl[])  [unwired: 9 in, 3 out]
        n92 = call "2nd_order_Poly_convert.vi"("Calib constants"=w350, "Voltage"=w344) -> ("Eng Values"=w352:dbl[])  [unwired: 4 out]
        n93 = Index Array(array=w352) -> (element=w351:dbl)  [unwired: 1 in]
        n94 = Replace Array Subset(array=w347, new element=w350, index=0) -> (w349:dbl[])
        n95 = Replace Array Subset(array=w349, new element=w351, index=3) -> (w348:dbl[])
      }
      frame "Single Hot wire" {
        n96 = Index Array(array=w390, index (col)=1) -> (element=w389:dbl[])  [unwired: 1 in]
        n97 = Index Array(array=w390, index (col)=0) -> (element=w388:dbl[])  [unwired: 1 in]
        n98 = Unbundle By Name(w405) -> ("Fraction"=w401:dbl)
        n99 = In Range and Coerce(upper limit=1.0, x=w401, lower limit=0.0) -> (coerced(x)=w387:dbl)  [unwired: 1 out]
        n100 = call "SingleWire_drift_correction_PN.vi"("calib consts. t1"=w394, "Tmeas (degC)"=w385, "variable n"=w384, "calib consts. t2"=w393, "{E_cal1}"=w389, "{U_cal1}"=w388, "time fraction"=w387, "wire diameter (mu.m)"=w383) -> ("[A, B, n]"=w386:dbl[])  [unwired: 1 in, 6 out]
        n101 = Build Array (concatenate)(w386, w385) -> (w395:dbl[])
        n102 = Format Into String(format string="Calib Fraction %.4f; ", initial string=w398, w387) -> (resulting string=w396:string)  [unwired: 1 in, 1 out]
        n103 = Replace Array Subset(array=w394, new element=w395, index=0) -> (w407:dbl[])
      }
      frame "Cross wire" {
        n104 = for {
          tunnel: w438 -> [w495]
          tunnel: w439 -> [w494]
          tunnel: [w493] -> w432 mode=indexing
          tunnel: [w492] -> w431 mode=indexing
          tunnel: i32[] [0, 1, 2, 9, 10, 12, 14, 15] -> [w491] mode=indexing
          n105 = Index Array(array=w495, index=w491) -> (element=w493:dbl)
          n106 = Index Array(array=w494, index=w491) -> (element=w492:dbl)
        }
        n107 = for {
          tunnel: i32[] [3, 4, 5, 9, 11, 13, 16, 17] -> [w490] mode=indexing
          tunnel: w439 -> [w489]
          tunnel: [w488] -> w424 mode=indexing
          tunnel: w438 -> [w487]
          tunnel: [w486] -> w425 mode=indexing
          n108 = Index Array(array=w487, index=w490) -> (element=w486:dbl)
          n109 = Index Array(array=w489, index=w490) -> (element=w488:dbl)
        }
        n110 = Index Array(array=w428, index (col)=1) -> (element=w430:dbl[])  [unwired: 1 in]
        n111 = Index Array(array=w428, index (col)=0) -> (element=w427:dbl[])  [unwired: 1 in]
        n112 = Index Array(array=w428, index (col)=2) -> (element=w426:dbl[])  [unwired: 1 in]
        n113 = Unbundle By Name(w452) -> ("Fraction"=w448:dbl)
        n114 = In Range and Coerce(upper limit=1.0, x=w448, lower limit=0.0) -> (coerced(x)=w423:dbl)  [unwired: 1 out]
        n115 = call "SingleWire_drift_correction_PN.vi"("calib consts. t1"=w432, "Tmeas (degC)"=w419, "variable n"=w420, "calib consts. t2"=w431, "{E_cal1}"=w430, "{U_cal1}"=w427, "time fraction"=w423, "wire diameter (mu.m)"=w418) -> ("[A, B, n]"=w422:dbl[])  [unwired: 1 in, 6 out]
        n116 = call "SingleWire_drift_correction_PN.vi"("calib consts. t1"=w425, "Tmeas (degC)"=w419, "variable n"=w420, "calib consts. t2"=w424, "{E_cal1}"=w426, "{U_cal1}"=w427, "time fraction"=w423, "wire diameter (mu.m)"=w418) -> ("[A, B, n]"=w421:dbl[])  [unwired: 1 in, 6 out]
        n117 = Replace Array Subset(array=w438, new element=w419, index=9) -> (w434:dbl[])
        n118 = Replace Array Subset(array=w434, new element=w422, index=0) -> (w433:dbl[])
        n119 = Replace Array Subset(array=w433, new element=w421, index=3) -> (w414:dbl[])
        n120 = Format Into String(format string="Calib Fraction %.4f; ", initial string=w445, w423) -> (resulting string=w443:string)  [unwired: 1 in, 1 out]
        n121 = case shown="False" w416 {
          tunnel: w417 -> [w461 _]
          tunnel: w415 -> [w455 _]
          tunnel: w414 -> [w460 _]
          tunnel: w413 -> [w459 _]
          tunnel: w412 -> [w458 _]
          tunnel: w411 -> [w457 _]
          tunnel: w410 -> [w456 _]
          frame False {
            n122 = case shown="\"Triangle mesh\", \"Polynomial surface\"" w455 {
              selector: w455 -> [w468 _ _]
              tunnel: w461 -> [w476 _ _]
              tunnel: w460 -> [w473 _ _]
              tunnel: w459 -> [w472 _ _]
              tunnel: w458 -> [w471 _ _]
              tunnel: w457 -> [w470 _ _]
              tunnel: w456 -> [w469 _ _]
              frame "Triangle mesh", "Polynomial surface" {
                n123 = Strip Path(path=w476) -> (stripped path=w465:path)  [unwired: 1 out]
                n124 = Build Path(base path=w465, name or relative path="XW_Map.txt") -> (appended path=w474:path)
                n125 = Build Path(base path=w465, name or relative path="XW_Map_CALPTS.txt") -> (appended path=w467:path)
                n126 = call "Does_file_exist_(simple).vi"("Pathname"=w474) -> ("exists?"=w463:bool)
                n127 = call "Does_file_exist_(simple).vi"("Pathname"=w467) -> ("exists?"=w464:bool)
                n128 = And(x=w463, y=w464) -> (x .and. y?=w462:bool)
                n129 = case shown="True" w462 {
                  tunnel: w474 -> [_ w483]
                  tunnel: w468 -> [_ w484]
                  tunnel: w473 -> [_ w482]
                  tunnel: w472 -> [_ w481]
                  tunnel: w471 -> [_ w480]
                  tunnel: w470 -> [_ w479]
                  tunnel: w469 -> [_ w478]
                  frame False {
                    n130 = global write "XW_Map_Global.vi" "Map method"(Map_method."Const. Psi_eff (std.)" ("Map method")) -> ()
                  }
                  frame True {
                    n131 = call "XW_Map_PreProc_wrapper_PN.vi"("Domain padding factor"=w478, "cap indicial sum to n"=w479, "XW_Calib_Map file path"=w483, "surface order (n)"=w480, "Apply calibration corrections"=w481, "Calib const"=w482, "Map method"=w484) -> ()  [unwired: 5 out]
                  }
                }
              }
              frame "Psi_eff = f(Umagn.)", "Psi_eff, k = f(Umagn.)" {
              }
              frame "Const. Psi_eff (std.)" {
                n132 = global write "XW_Map_Global.vi" "Map method"(Map_method."Const. Psi_eff (std.)" ("Map method")) -> ()
              }
            }
          }
          frame True {
          }
        }
      }
      frame "Bkgnd info from header" {
        # "Start"
        # "end"
        n133 = stacked-sequence {
          seq-local: [w515 _ _ _ _ _ _] -> [_ _ w536 _ w657 _ _]
          seq-local: [w517 _ _ _ _ _ _] -> [_ _ w534 _ w649 _ _]
          seq-local: [w516 _ _ _ _ _ _] -> [_ _ w533 _ w660 _ _]
          seq-local: [_ w524 _ _ _ _ _] -> [_ _ w532 _ w658 w837 _]
          seq-local: [_ _ w531 _ _ _ _] -> [_ _ _ _ w655 _ _]
          seq-local: [_ _ w530 _ _ _ _] -> [_ _ _ w646 w659 w838 _]
          seq-local: [_ _ w529 _ _ _ _] -> [_ _ _ w647 _ w839 _]
          seq-local: [_ _ _ w632 _ _ _] -> [_ _ _ _ w662 _ _]
          seq-local: [_ _ _ w641 _ _ _] -> [_ _ _ _ _ w840 _]
          seq-local: [_ _ _ _ w652 _ _] -> [_ _ _ _ _ w834 _]
          tunnel: w514 -> [w518 w523 _ _ _ _ _]
          tunnel: w513 -> [_ _ w535 _ w650 _ _]
          tunnel: w512 -> [_ w519 _ w648 _ w836 _]
          tunnel: [_ w523 _ _ _ _ _] -> w511
          tunnel: w510 -> [_ w522 _ _ _ _ _]
          tunnel: [_ w522 _ _ _ _ _] -> w509
          tunnel: [_ w521 _ _ _ _ _] -> w508
          tunnel: w507 -> [_ w521 _ _ _ _ _]
          tunnel: w506 -> [_ _ _ _ w656 w835 _]
          tunnel: [_ _ _ _ _ w833 _] -> w505
          tunnel: [_ w520 _ _ _ _ _] -> w504
          tunnel: w503 -> [_ w520 _ _ _ _ _]
          tunnel: [_ _ _ _ _ _ w899] -> w502
          tunnel: [_ _ _ _ TRUE _ _] -> w501
          tunnel: [_ w519 _ _ _ _ _] -> w500
          tunnel: [_ _ _ _ w653 _ _] -> w499
          tunnel: w498 -> [_ _ _ _ w654 _ _]
          tunnel: w496 -> [_ _ _ _ w661 _ w901]
          frame #0 {
            n134 = call "Read FFID_Header.vi"("Raw Data header String"=w518) -> ("Ch names"=w517:string[], "FFID Header Info"=w516:string[][], "Bkgnd Volts Present?"=w515:bool)
            "Header info" <- w516
          }
          frame #1 {
            n135 = Unbundle By Name(w519) -> ("Meas start time"=w528:dbl, "Meas end time"=w527:dbl)
            n136 = Add(x=w528, y=w527) -> (x+y=w526:dbl)
            n137 = Divide(x=w526, y=2.0) -> (x/y=w524:dbl)
          }
          frame #2 {
            n138 = case shown="True" w536 {
              tunnel: w535 -> [w554 w608]
              tunnel: w534 -> [w541 w598]
              tunnel: w533 -> [w543 w599]
              tunnel: w532 -> [w540 _]
              tunnel: [w539 w585] -> w531
              tunnel: [w538 w585] -> w530
              tunnel: [w537 w585] -> w529
              frame True {
                n139 = Decimal String To Number(string=w554) -> (number=w553:i32)  [unwired: 3 out]
                n140 = Index Array(array=w543, index (col)=0 ("disabled index (col)")) -> (element=w548:string[])  [unwired: 1 in]
                n141 = Number To Decimal String(number=w553) -> (decimal integer string=w552:string)  [unwired: 1 out]
                n142 = Search 1D Array(1D array=w548, element="Calibration Before Meas") -> (index of element=w546:i32)  [unwired: 1 out]
                n143 = Search 1D Array(1D array=w548, element="Calibration After Meas") -> (index of element=w544:i32)  [unwired: 1 out]
                n144 = Index Array(array=w543, index (row)=w546) -> (element=w545:string[])  [unwired: 1 in]
                n145 = Index Array(array=w543, index (row)=w544) -> (element=w542:string[])  [unwired: 1 in]
                n146 = for {
                  tunnel: w552 -> [w570]
                  tunnel: string[] ["Bkgnd Time", "Bkgnd Volts", "Bkgnd Variance"] ("appended array") -> [w569] mode=indexing
                  tunnel: w545 -> [w568]
                  tunnel: w542 -> [w566]
                  tunnel: w541 -> [w564]
                  tunnel: w540 -> [w562]
                  shift-right: [w558] -> _
                  shift-left: _ -> [w559]
                  tunnel: [w557] -> w539 mode=indexing
                  tunnel: [w556] -> w538 mode=indexing
                  tunnel: [w555] -> w537 mode=indexing
                  i -> [w563]
                  # "After"
                  # "Before"
                  n147 = Concatenate Strings("FF:", w570, ":" ("Substring"), w569) -> (w571:string)
                  n148 = Search 1D Array(1D array=w564, element=w571) -> (index of element=w567:i32)  [unwired: 1 out]
                  n149 = Index Array(array=w568, index=w567) -> (element=w561:string)
                  n150 = Index Array(array=w566, index=w567) -> (element=w560:string)
                  n151 = call "String_2_Number.vi"("Value"=w561) -> ("Numeric"=w556:dbl)
                  n152 = call "String_2_Number.vi"("Value"=w560) -> ("Numeric"=w555:dbl)
                  n153 = case shown="1, Default" w563 {
                    tunnel: w562 -> [w578 _]
                    tunnel: w556 -> [w576 w581]
                    tunnel: w555 -> [w577 w584]
                    tunnel: [w573 w580] -> w557
                    tunnel: w559 -> [_ w579]
                    tunnel: [w573 w579] -> w558
                    frame 0 {
                      n154 = Subtract(x=w578, y=w576) -> (x-y=w574:dbl)
                      n155 = Subtract(x=w577, y=w576) -> (x-y=w575:dbl)
                      n156 = Divide(x=w574, y=w575) -> (x/y=w573:dbl)
                    }
                    frame 1, Default {
                      n157 = Subtract(x=w584, y=w581) -> (x-y=w583:dbl)
                      n158 = Multiply(x=w579, y=w583) -> (x*y=w582:dbl)
                      n159 = Add(x=w582, y=w581) -> (x+y=w580:dbl)
                    }
                  }
                }
              }
              frame False {
                n160 = Decimal String To Number(string=w608) -> (number=w607:i32)  [unwired: 3 out]
                n161 = Index Array(array=w599, index (col)=0 ("disabled index (col)")) -> (element=w602:string[])  [unwired: 1 in]
                n162 = Number To Decimal String(number=w607) -> (decimal integer string=w606:string)  [unwired: 1 out]
                n163 = Search 1D Array(1D array=w602, element="Calibration To be Used") -> (index of element=w601:i32)  [unwired: 1 out]
                n164 = Index Array(array=w599, index (row)=w601) -> (element=w600:string[])  [unwired: 1 in]
                n165 = for {
                  tunnel: w606 -> [w629]
                  tunnel: string[] ["Coeff A", "Coeff B", "Coeff C", "Bkgnd", "Bkgnd Variance"] ("appended array") -> [w628] mode=indexing
                  tunnel: w600 -> [w627]
                  tunnel: w598 -> [w625]
                  tunnel: [w623] -> w588 mode=indexing
                  tunnel: [w622] -> w591 mode=indexing
                  n166 = Concatenate Strings("FF:", w629, ":" ("Substring"), w628) -> (w630:string)
                  n167 = Search 1D Array(1D array=w625, element=w630) -> (index of element=w622:i32)  [unwired: 1 out]
                  n168 = Index Array(array=w627, index=w622) -> (element=w624:string)
                  n169 = call "String_2_Number.vi"("Value"=w624) -> ("Numeric"=w623:dbl)
                }
                n170 = Index Array(array=w588, index=3 ("length")) -> (element=w596:dbl)
                n171 = Index Array(array=w588, index=4) -> (element=w593:dbl)
                n172 = Index Array(array=w591, index=2) -> (element=w589:i32)
                n173 = Less Than 0?(x=w589) -> (x < 0?=w587:bool)
                n174 = case shown="False" w587 {
                  tunnel: w588 -> [w610 w616]
                  tunnel: [w609 w612] -> w586
                  frame False {
                    n175 = Array Subset(array=w610, length=3) -> (w609:dbl[])  [unwired: 1 in]
                  }
                  frame True {
                    n176 = Index Array(array=w616, index=1) -> (element=w620:dbl)
                    n177 = Index Array(array=w616, index=0) -> (element=w619:dbl)
                    n178 = Reciprocal(x=w620) -> (1/x=w614:dbl)
                    n179 = Divide(x=w619, y=w620) -> (x/y=w621:dbl)
                    n180 = Negate(x=w621) -> (-x=w615:dbl)
                    n181 = Build Array(w615, w614, 0.0 ("element")) -> (w612:dbl[])
                  }
                }
                n182 = call "Polybackwards.vi"("Coefficients"=w586, "Y input"=w596) -> ("X output"=w594:dbl)  [unwired: 1 out]
                n183 = Build Array(0.0 ("element"), w594, w593) -> (w585:dbl[])
              }
            }
          }
          frame #3 {
            # "Bkgnd Time"
            n184 = Unbundle By Name(w648) -> ("1st Calib time"=w640:dbl, "2nd Calib time"=w635:dbl)
            n185 = Index Array(array=w647) -> (element #1=w636:dbl, element #2=w638:dbl)  [unwired: 2 in]
            n186 = Index Array(array=w646) -> (element #1=w645:dbl, element #2=w639:dbl)  [unwired: 2 in]
            n187 = Greater?(x=w636, y=w635) -> (0:w633:bool)
            n188 = Greater Than 0?(x=w635) -> (x > 0?=w634:bool)
            n189 = Greater?(x=w639, y=w638) -> (0:w642:bool)
            n190 = And(x=w633, y=w634) -> (x .and. y?=w632:bool)
            n191 = Subtract(x=w645, y=w640) -> (x-y=w637:dbl)
            n192 = Less?(x=w637, y=250.0) -> (x < y?=w643:bool)
            n193 = And(x=w643, y=w642) -> (x .and. y?=w641:bool)
          }
          frame #4 {
            n194 = case shown="True" w662 {
              tunnel: w661 -> [_ w726]
              tunnel: w660 -> [_ w725]
              tunnel: w659 -> [w669 w724]
              tunnel: w658 -> [_ w723]
              tunnel: w657 -> [w668 _]
              tunnel: w656 -> [w667 w720]
              tunnel: w655 -> [w666 w722]
              tunnel: w654 -> [w665 w719]
              tunnel: [w664 w718] -> w653
              tunnel: [w663 w721] -> w652
              tunnel: w650 -> [_ w717]
              tunnel: w649 -> [_ w716]
              frame False {
                n195 = Index Array(array=w666, index=1) -> (element=w672:dbl)
                n196 = Index Array(array=w666, index=2) -> (element=w679:dbl)
                n197 = Build Array(w672) -> (w671:dbl[])
                n198 = Index Array(array=w669) -> (element #1=w675:dbl, element #2=w674:dbl, element #3=w673:dbl)  [unwired: 3 in]
                n199 = Index Array(array=w666, index=0) -> (element=w677:dbl)
                n200 = call "2nd_order_Poly_convert.vi"("Calib constants"=w667, "Voltage"=w671) -> ("Eng Values"=w684:dbl[])  [unwired: 4 out]
                n201 = Not A Number/Path/Refnum?(number/path/refnum=w666) -> (NaN/Path/Refnum?=w676:bool[])
                n202 = Or Array Elements(Boolean array=w676) -> (logical OR=w670:bool)
                n203 = Index Array(array=w684, index=0) -> (element=w680:dbl)
                n204 = case shown="False" w670 {
                  tunnel: w667 -> [w702 w714]
                  tunnel: w680 -> [w700 _]
                  tunnel: w679 -> [w697 _]
                  tunnel: [w688 w714] -> w663
                  tunnel: w677 -> [w695 _]
                  tunnel: [w692 w715] -> w664
                  tunnel: w665 -> [w691 w715]
                  tunnel: w668 -> [w685 _]
                  tunnel: w675 -> [w690 _]
                  tunnel: w674 -> [w687 _]
                  tunnel: w673 -> [w686 _]
                  frame False {
                    n205 = Equal To 0?(x=w695) -> (x = 0?=w694:bool)
                    n206 = Replace Array Subset(array=w702, new element=w700, index=3) -> (w699:dbl[])
                    n207 = Format Into String(format string="Bkgnd Fraction %.4f; ", initial string=w691, w695) -> (resulting string=w693:string)  [unwired: 1 in, 1 out]
                    n208 = Replace Array Subset(array=w699, new element=w697, index=4) -> (w689:dbl[])
                    n209 = case shown="True" w685 {
                      tunnel: w690 -> [_ w713]
                      tunnel: w689 -> [w703 w712]
                      tunnel: [w703 w707] -> w688
                      tunnel: w687 -> [_ w706]
                      tunnel: w686 -> [_ w705]
                      frame False {
                      }
                      frame True {
                        n210 = Replace Array Subset(array=w712, new element=w713, index=8) -> (w709:dbl[])
                        n211 = Replace Array Subset(array=w709, new element=w706, index=9) -> (w708:dbl[])
                        n212 = Replace Array Subset(array=w708, new element=w705, index=10) -> (w707:dbl[])
                      }
                    }
                    n213 = Select(t=w691, s=w694, f=w693) -> (s? t:f=w692:string)
                  }
                  frame True {
                  }
                }
              }
              frame True {
                # "File"
                # "Time"
                # "Volts"
                n214 = stacked-sequence {
                  seq-local: [_ w745 _ _] -> [_ _ w812 _]
                  seq-local: [_ w744 _ _] -> [_ _ w811 _]
                  seq-local: [_ w743 _ _] -> [_ _ _ w819]
                  seq-local: [_ _ w792 _] -> [_ _ _ w813]
                  seq-local: [w731 _ _ _] -> [_ w742 _ _]
                  seq-local: [w727 _ _ _] -> [_ w741 _ _]
                  tunnel: w726 -> [_ w762 _ _]
                  tunnel: w725 -> [_ w748 _ w821]
                  tunnel: w724 -> [_ _ w810 _]
                  tunnel: w723 -> [_ _ w795 _]
                  tunnel: w722 -> [_ _ _ _]
                  tunnel: [_ _ _ w816] -> w721
                  tunnel: w720 -> [_ _ w798 w817]
                  tunnel: w719 -> [_ _ _ w815]
                  tunnel: [_ _ _ w814] -> w718
                  tunnel: w717 -> [w734 _ _ _]
                  tunnel: w716 -> [w728 _ _ _]
                  frame #0 {
                    n215 = Decimal String To Number(string=w734) -> (number=w735:i32)  [unwired: 3 out]
                    n216 = Number To Decimal String(number=w735) -> (decimal integer string=w732:string)  [unwired: 1 out]
                    n217 = for {
                      tunnel: string[] ["Calib Filename", "Bkgnd Volts", "Bkgnd Time"] ("appended array") -> [w738] mode=indexing
                      tunnel: w732 -> [w737]
                      tunnel: [w736] -> w731 mode=indexing
                      n218 = Concatenate Strings("FF:", w737, ":" ("Substring"), w738) -> (w736:string)
                    }
                    n219 = Index Array(array=w731, index=2) -> (element=w729:string)
                    n220 = Search 1D Array(1D array=w728, element=w729) -> (index of element=w727:i32)  [unwired: 1 out]
                  }
                  frame #1 {
                    w754 = "_" ("regular expression")
                    n221 = Index Array(array=w748, index (row)=0, index (col)=w741) -> (element=w747:string)
                    n222 = Strip Path(path=w762) -> (stripped path=w746:path, name=w761:string)
                    n223 = Reverse String(1:w761) -> (0:w760:string)
                    n224 = Match Pattern(string=w760, regular expression=w754) -> (before substring=w759:string, after substring=w756:string)  [unwired: 1 in, 2 out]
                    n225 = Reverse String(1:w759) -> (0:w757:string)
                    n226 = Reverse String(1:w756) -> (0:w755:string)
                    n227 = Decimal String To Number(string=w757) -> (offset past number=w758:i32, number=w751:i32)  [unwired: 2 in]
                    n228 = Decrement(x=w751) -> (x-1=w750:i32)
                    n229 = String Subset(string=w757, offset (0)=w758) -> (substring=w753:string)  [unwired: 1 in]
                    n230 = for {
                      N: 20 -> [_]
                      tunnel: w755 -> [w785]
                      tunnel: w754 -> [w784]
                      tunnel: w753 -> [w782]
                      tunnel: w750 -> [w780]
                      tunnel: w747 -> [w773]
                      tunnel: w746 -> [w771]
                      tunnel: [w764] -> w745
                      tunnel: [w763] -> w744
                      tunnel: [w765] -> w743
                      tunnel: w742 -> [w768]
                      i -> [w781]
                      stop <- w772 continue-if-true
                      w776 = FALSE  # Show Dialog?
                      n231 = Subtract(x=w780, y=w781) -> (x-y=w779:i32)
                      n232 = Number To Decimal String(number=w779) -> (decimal integer string=w783:string)  [unwired: 1 in]
                      n233 = Concatenate Strings(w785, w784, w783, w782) -> (w770:string)
                      "Earlier raw data file" <- w770
                      n234 = Build Path(base path=w771, name or relative path=w770) -> (appended path=w778:path)
                      n235 = Read from Text File(file (use dialog)=w778) -> (text=w775:string)  [unwired: 3 in, 3 out]
                      n236 = call "Get_string_subset.vi"("Show Dialog?"=w776, "String to split"=w775, "File Label"="Raw data header") -> ("Output string"=w774:string)  [unwired: 1 in, 1 out]
                      n237 = call "Read FFID_Header.vi"("Raw Data header String"=w774) -> ("Ch names"=w769:string[], "FFID Header Info"=w767:string[][])  [unwired: 1 out]
                      n238 = for {
                        tunnel: [w790] -> w766 mode=indexing
                        tunnel: w769 -> [w789]
                        tunnel: w768 -> [w787] mode=indexing
                        tunnel: w767 -> [w786]
                        n239 = Search 1D Array(1D array=w789, element=w787) -> (index of element=w788:i32)  [unwired: 1 out]
                        n240 = Index Array(array=w786, index (row)=0, index (col)=w788) -> (element=w790:string)
                      }
                      n241 = Index Array(array=w766) -> (element #1=w765:string, element #2=w764:string, element #3=w763:string)  [unwired: 3 in]
                      n242 = Equal?(x=w763, y=w773) -> (x = y?=w772:bool)
                    }
                  }
                  frame #2 {
                    n243 = Index Array(array=w810) -> (element #1=w809:dbl, element #2=w807:dbl)  [unwired: 2 in]
                    n244 = Fract/Exp String To Number(string=w812) -> (number=w808:dbl)  [unwired: 3 in, 1 out]
                    "Volts" <- w808
                    n245 = Fract/Exp String To Number(string=w811) -> (number=w794:dbl)  [unwired: 3 in, 1 out]
                    "Time" <- w794
                    n246 = Build Array(w794, w809) -> (w797:dbl[])
                    n247 = Subtract(x=w797, y=w794) -> (x-y=w796:dbl[])
                    n248 = Build Array(w808, w807) -> (w806:dbl[])
                    n249 = Subtract(x=w795, y=w794) -> (x-y=w793:dbl)
                    n250 = call <vilib>:"Linear Fit.vi"("Y"=w806, "X"=w796) -> ("slope"=w805:dbl, "intercept"=w803:dbl)  [unwired: 9 in, 3 out]
                    n251 = Multiply(x=w793, y=w805) -> (x*y=w804:dbl)
                    n252 = Add(x=w804, y=w803) -> (x+y=w799:dbl)
                    n253 = Build Array(w799) -> (w800:dbl[])
                    n254 = call "2nd_order_Poly_convert.vi"("Calib constants"=w798, "Voltage"=w800) -> ("Eng Values"=w802:dbl[])  [unwired: 4 out]
                    n255 = Index Array(array=w802, index=0) -> (element=w792:dbl)
                  }
                  frame #3 {
                    n256 = Index Array(array=w821, index (row)=0, index (col)=1 ("disabled index (col)")) -> (element=w820:string)
                    n257 = Equal?(x=w819, y=w820) -> (x = y?=w818:bool)
                    n258 = case shown="True" w818 {
                      tunnel: w817 -> [w825 w831]
                      tunnel: [w825 w830] -> w816
                      tunnel: w815 -> [w824 w829]
                      tunnel: [w824 w828] -> w814
                      tunnel: w813 -> [_ w826]
                      frame False {
                      }
                      frame True {
                        n259 = Replace Array Subset(array=w831, new element=w826, index=3) -> (w830:dbl[])
                        n260 = Concatenate Strings(w829, "Bkgnd Extrapolated;" ("string")) -> (w828:string)
                      }
                    }
                  }
                }
              }
            }
          }
          frame #5 {
            n261 = case shown="True" w840 {
              tunnel: w839 -> [_ w854]
              tunnel: w838 -> [_ w853]
              tunnel: w837 -> [_ w847]
              tunnel: w836 -> [_ w846]
              tunnel: w835 -> [_ w844]
              tunnel: w834 -> [w841 w843]
              tunnel: [w841 w842] -> w833
              frame False {
              }
              frame True {
                w850 = 350.0  # Time Constant
                # "Offset"
                # "A"
                # "B2"
                # "B1"
                # "T2"
                # "T1"
                # "Ratio 2"
                # "Ratio 1"
                n262 = Unbundle By Name(w846) -> ("1st Calib time"=w845:dbl)
                n263 = Index Array(array=w854) -> (element #1=w851:dbl, element #2=w848:dbl)  [unwired: 2 in]
                n264 = Index Array(array=w853) -> (element #1=w852:dbl, element #2=w849:dbl)  [unwired: 2 in]
                n265 = stacked-sequence {
                  seq-local: [w865 _ _ _ _] -> [_ w871 _ _ _]
                  seq-local: [w863 _ _ _ _] -> [_ w870 w876 _ _]
                  seq-local: [_ w867 _ _ _] -> [_ _ w875 w882 _]
                  seq-local: [_ _ w877 _ _] -> [_ _ _ w880 _]
                  seq-local: [_ _ _ w879 _] -> [_ _ _ _ w894]
                  tunnel: w852 -> [w859 _ _ _ _]
                  tunnel: w851 -> [w856 _ _ _ _]
                  tunnel: w850 -> [w860 _ _ w887 _]
                  tunnel: w849 -> [_ w873 _ _ _]
                  tunnel: w848 -> [_ w872 w878 _ _]
                  tunnel: w847 -> [_ _ _ w885 _]
                  tunnel: w845 -> [w857 _ _ w886 _]
                  tunnel: w844 -> [_ _ _ _ w893]
                  tunnel: w843 -> [_ _ _ _ w892]
                  tunnel: [_ _ _ _ w891] -> w842
                  frame #0 {
                    n266 = Subtract(x=w859, y=w857) -> (x-y=w858:dbl)
                    n267 = Subtract(x=w856, y=w857) -> (x-y=w855:dbl)
                    n268 = Divide(x=w858, y=w860) -> (x/y=w866:dbl)
                    n269 = Divide(x=w855, y=w860) -> (x/y=w864:dbl)
                    n270 = Negate(x=w866) -> (-x=w862:dbl)
                    n271 = Negate(x=w864) -> (-x=w861:dbl)
                    n272 = Exponential(1:w862) -> (0:w865:dbl)
                    n273 = Exponential(1:w861) -> (0:w863:dbl)
                  }
                  frame #1 {
                    n274 = Subtract(x=w871, y=w870) -> (x-y=w868:dbl)
                    n275 = Subtract(x=w873, y=w872) -> (x-y=w869:dbl)
                    n276 = Divide(x=w869, y=w868) -> (x/y=w867:dbl)
                  }
                  frame #2 {
                    n277 = Multiply(x=w876, y=w875) -> (x*y=w874:dbl)
                    n278 = Subtract(x=w878, y=w874) -> (x-y=w877:dbl)
                  }
                  frame #3 {
                    n279 = Subtract(x=w885, y=w886) -> (x-y=w884:dbl)
                    n280 = Divide(x=w884, y=w887) -> (x/y=w888:dbl)
                    n281 = Negate(x=w888) -> (-x=w889:dbl)
                    n282 = Exponential(1:w889) -> (0:w883:dbl)
                    n283 = Multiply(x=w882, y=w883) -> (x*y=w881:dbl)
                    n284 = Add(x=w881, y=w880) -> (x+y=w879:dbl)
                  }
                  frame #4 {
                    n285 = Build Array(w894) -> (w898:dbl[])
                    n286 = call "2nd_order_Poly_convert.vi"("Calib constants"=w893, "Voltage"=w898) -> ("Eng Values"=w897:dbl[])  [unwired: 4 out]
                    n287 = Index Array(array=w897, index=0) -> (element=w890:dbl)
                    n288 = Replace Array Subset(array=w892, new element=w890, index=3) -> (w891:dbl[])
                  }
                }
              }
            }
          }
          frame #6 {
            n289 = Strip Path(path=w901) -> (stripped path=w905:path)  [unwired: 1 out]
            n290 = Build Path(base path=w905, name or relative path="Background_History.xls") -> (appended path=w904:path)
            n291 = call "Does_file_exist_(simple).vi"("Pathname"=w904) -> ("exists?"=w903:bool)
            n292 = Select(t="Bkgnd info from table", s=w903, f="Add FFID Bkgnd Values") -> (s? t:f=w899:string)
          }
        }
      }
      frame "Bkgnd info from table" {
        n293 = stacked-sequence {
          seq-local: [w940 _] -> [_ w952]
          seq-local: [_ w966] -> [_ _]
          seq-local: [w941 _] -> [_ w967]
          seq-local: [w939 _] -> [_ w944]
          tunnel: w924 -> [_ w975]
          tunnel: w923 -> [_ w970]
          tunnel: w922 -> [_ w971]
          tunnel: [_ w975] -> w921
          tunnel: w920 -> [_ w974]
          tunnel: [_ w974] -> w919
          tunnel: [_ w973] -> w918
          tunnel: w917 -> [_ w973]
          tunnel: w916 -> [_ w958]
          tunnel: [_ w948] -> w915
          tunnel: [_ w972] -> w914
          tunnel: w913 -> [_ w972]
          tunnel: [_ "Add FFID Bkgnd Values"] -> w912
          tunnel: [_ TRUE] -> w911
          tunnel: [_ w971] -> w910
          tunnel: w909 -> [_ w954]
          tunnel: [_ w953] -> w908
          frame #0 {
            n294 = global read "Meas_global.vi" "Raw data file"() -> (w938:path)
            n295 = Strip Path(path=w938) -> (stripped path=w936:path)  [unwired: 1 out]
            n296 = Build Path(base path=w936, name or relative path="Background_History.xls") -> (appended path=w935:path)
            n297 = call "Read_File_Simple.vi"("Filename"=w935) -> ("string"=w934:string)  [unwired: 2 in, 7 out]
            n298 = call "String_to_Ch_names.vi"("Spreadsheet string"=w934) -> ("Ch names"=w926:string[], "String After names"=w931:string)  [unwired: 2 out]
            n299 = Spreadsheet String To Array(format string="%s", spreadsheet string=w931, array type (2D Dbl)=string[][] []) -> (array=w928:string[][])  [unwired: 1 out]
            n300 = Search 1D Array(1D array=w926, element="Seconds:since:1st Jan") -> (index of element=w927:i32)  [unwired: 1 out]
            n301 = Increment(x=w927) -> (x+1=w925:i32)
            n302 = Index Array(array=w928, index (col)=w927) -> (element=w929:string[])  [unwired: 1 in]
            n303 = Array Subset(array=w928, index (col)=w925) -> (w940:string[][])  [unwired: 3 in]
            n304 = call "String_2_Number_array.vi"("Input String"=w929) -> ("Values"=w941:dbl[])
            n305 = Array Subset(array=w926, index=w925) -> (w939:string[])  [unwired: 1 in]
          }
          frame #1 {
            n306 = Unbundle By Name(w971) -> ("Meas start time"=w979:dbl, "Meas end time"=w978:dbl)
            n307 = Decimal String To Number(string=w970) -> (number=w946:i32)  [unwired: 3 out]
            n308 = Format Into String(format string="FF:%d:Bkgnd c^2", w946) -> (resulting string=w945:string)  [unwired: 2 in, 1 out]
            n309 = Search 1D Array(1D array=w944, element=w945) -> (index of element=w943:i32)  [unwired: 1 in]
            n310 = Decrement(x=w946) -> (x-1=w969:i32)
            n311 = Add(x=w979, y=w978) -> (x+y=w977:dbl)
            n312 = Divide(x=w977, y=2.0) -> (x/y=w966:dbl)
            n313 = Index Array(array=w952, index (col)=w969) -> (element=w968:string[])  [unwired: 1 in]
            n314 = Threshold 1D Array(2:w966, 3:w967) -> (0:w951:dbl)  [unwired: 1 out]
            n315 = case shown="1, Default" w943 {
              tunnel: w952 -> [_ w988]
              tunnel: w951 -> [_ w983]
              tunnel: [0.22 w985] -> w947
              tunnel: w943 -> [_ w984]
              frame -1 {
              }
              frame 1, Default {
                n316 = Index Array(array=w988, index (col)=w984) -> (element=w987:string[])  [unwired: 1 in]
                n317 = call "String_2_Number_array.vi"("Input String"=w987) -> ("Values"=w986:dbl[])
                n318 = Interpolate 1D Array(1:w983, 2:w986) -> (0:w985:dbl)
              }
            }
            n319 = for {
              tunnel: w968 -> [w981] mode=indexing
              tunnel: [w980] -> w965 mode=indexing
              n320 = call "String_2_Number.vi"("Value"=w981) -> ("Numeric"=w980:dbl)
            }
            n321 = Interpolate 1D Array(1:w951, 2:w965) -> (0:w957:dbl)
            n322 = Build Array(w957) -> (w961:dbl[])
            n323 = Format Into String(format string="Bkgnd Index %.2f; ", initial string=w954, w951) -> (resulting string=w953:string)  [unwired: 1 in, 1 out]
            n324 = call "2nd_order_Poly_convert.vi"("Calib constants"=w958, "Voltage"=w961) -> ("Eng Values"=w960:dbl[])  [unwired: 4 out]
            n325 = Index Array(array=w960, index=0) -> (element=w956:dbl)
            n326 = Replace Array Subset(array=w958, new element=w956, index=3) -> (w949:dbl[])
            n327 = Replace Array Subset(array=w949, new element=w947, index=4) -> (w948:dbl[])
          }
        }
      }
      frame "Add FFID Bkgnd Values" {
        n328 = global read "Plug_in_data_global.vi" "FFID Bkgnd Values"() -> (w995:dbl[])
        n329 = global read "Dynamic_call_global.ph.vi" "Per Block Plug Ins"() -> (w994:string[])
        n330 = Array Size(array=w995) -> (size(s)=w1002:i32)
        n331 = Search 1D Array(1D array=w994, element="Puff_Dose.vi") -> (index of element=w992:i32)  [unwired: 1 in]
        n332 = Greater Than 0?(x=w1002) -> (x > 0?=w990:bool)
        n333 = Less Than 0?(x=w992) -> (x < 0?=w991:bool)
        n334 = And(x=w990, y=w991) -> (x .and. y?=w989:bool)
        n335 = case shown="True" w989 {
          tunnel: w1001 -> [w1010 w1025]
          tunnel: [w1010 w1024] -> w1000
          tunnel: w995 -> [_ w1019]
          tunnel: w999 -> [w1009 w1020]
          tunnel: [w1009 w1018] -> w998
          frame False {
          }
          frame True {
            # "20 blocks of 3 sec bkgnd"
            n336 = Index Array(array=w1019, index=0) -> (element=w1017:dbl)
            n337 = Not A Number/Path/Refnum?(number/path/refnum=w1017) -> (NaN/Path/Refnum?=w1016:bool)
            n338 = case shown="False" w1016 {
              tunnel: w1025 -> [w1028 w1030]
              tunnel: [w1027 w1030] -> w1024
              tunnel: w1017 -> [w1026 _]
              frame False {
                n339 = Replace Array Subset(array=w1028, new element=w1026, index=3) -> (w1027:dbl[])
              }
              frame True {
              }
            }
            n340 = Index Array(array=w1019, index=1) -> (element=w1014:dbl)
            n341 = Index Array(array=w1019, index=2) -> (element=w1012:dbl)
            n342 = Array Subset(array=w1019, index=3) -> (w1021:dbl[])  [unwired: 1 in]
            n343 = global write "Plug_in_data_global.vi" "FFID Bkgnd Values"(w1021) -> ()
            n344 = Format Into String(format string="%d blocks of %d Sec Bkgnd; ", initial string=w1020, w1014, w1012) -> (resulting string=w1018:string)  [unwired: 1 in, 1 out]
          }
        }
      }
      frame "Add Drift Info" {
        n345 = call "Get_Characters_from_string.vi"("Show Dialog?"=FALSE, "Input string"=w1042, "Variable name"="Percentage Drift till Next calibration") -> ("Status"=w1049:enum16{"Char in string", "Char not in string"}, "Value"=w1050:string)
        n346 = Empty String/Path?(string/path=w1038) -> (empty?=w1037:bool)
        n347 = case shown="True" w1037 {
          tunnel: w1038 -> [w1083 _]
          tunnel: w1032 -> [w1081 w1085]
          tunnel: [w1078 w1085] -> w1031
          frame False {
            n348 = Unbundle By Name(w1081) -> ("Extra Titles"=w1082:string[], "Extra Values"=w1084:string[])
            n349 = Build Array (concatenate)(w1084, w1083) -> (w1079:string[])
            n350 = Build Array (concatenate)(w1082, "Correction:Info" ("string")) -> (w1080:string[])
            n351 = Bundle By Name(cluster=w1081, "Extra Titles"=w1080, "Extra Values"=w1079) -> (w1078:T1)
          }
          frame True {
          }
        }
        n352 = case shown="\"Char not in string\"" w1049 {
          tunnel: [w1092 nan ("Value")] -> w1041
          tunnel: w1050 -> [w1088 _]
          frame "Char in string" {
            n353 = Match Pattern(string=w1088, regular expression="Drift_Place_Holder") -> (offset past match=w1090:i32)  [unwired: 4 out]
            n354 = Greater Than 0?(x=w1090) -> (x > 0?=w1089:bool)
            n355 = case shown="False" w1089 {
              tunnel: [w1093 nan ("Value")] -> w1092
              tunnel: w1088 -> [w1094 _]
              frame False {
                n356 = call "String_2_Number.vi"("Value"=w1094) -> ("Numeric"=w1093:dbl)
              }
              frame True {
              }
            }
          }
          frame "Char not in string" {
          }
        }
        n357 = call "Get_value_from_string.vi"("Show Dialog?"=FALSE, "Input string"=w1042, "Variable name"="Minutes Until Next calibration") -> ("Status"=w1045:enum16{"Char in string", "Char not in string"}, "Value"=w1046:dbl)
        n358 = Array Size(array=w1051) -> (size(s)=w1052:i32)
        n359 = case shown="\"Char not in string\"" w1045 {
          tunnel: [w1086 nan ("Value")] -> w1040
          tunnel: w1046 -> [w1086 _]
          frame "Char in string" {
          }
          frame "Char not in string" {
          }
        }
        n360 = Subtract(x=18, y=w1052) -> (x-y=w1054:i32)
        n361 = Initialize Array(0.0 ("Element Data"), w1054) -> (w1056:dbl[])
        n362 = Build Array (concatenate)(w1051, w1056, w1041, w1040) -> (w1036:dbl[])
        n363 = case shown="False" w1034 {
          tunnel: w1035 -> [w1063 _]
          tunnel: w1033 -> [w1062 _]
          frame False {
            n364 = case shown="\"Psi_eff = f(Umagn.)\", \"Psi_eff, k = f(Umagn.)\"" w1062 {
              selector: w1062 -> [_ w1070 _]
              tunnel: w1063 -> [_ w1073 _]
              frame "Triangle mesh", "Polynomial surface" {
              }
              frame "Psi_eff = f(Umagn.)", "Psi_eff, k = f(Umagn.)" {
                n365 = Strip Path(path=w1073) -> (stripped path=w1068:path)  [unwired: 1 out]
                n366 = Build Path(base path=w1068, name or relative path="XW_Map.txt") -> (appended path=w1071:path)
                n367 = Build Path(base path=w1068, name or relative path="XW_Map_CALPTS.txt") -> (appended path=w1067:path)
                n368 = call "Does_file_exist_(simple).vi"("Pathname"=w1071) -> ("exists?"=w1066:bool)
                n369 = call "Does_file_exist_(simple).vi"("Pathname"=w1067) -> ("exists?"=w1065:bool)
                n370 = And(x=w1066, y=w1065) -> (x .and. y?=w1064:bool)
                n371 = case shown="True" w1064 {
                  tunnel: w1070 -> [_ w1075]
                  frame False {
                    n372 = global write "XW_Map_Global.vi" "Map method"(Map_method."Const. Psi_eff (std.)" ("Map method")) -> ()
                  }
                  frame True {
                    n373 = call "XW_Higher_order_Psi_k_PreProc_PN.vi"("Map method"=w1075) -> ()  [unwired: 1 in, 1 out]
                  }
                }
              }
              frame "Const. Psi_eff (std.)" {
                n374 = global write "XW_Map_Global.vi" "Map method"(Map_method."Const. Psi_eff (std.)" ("Map method")) -> ()
              }
            }
          }
          frame True {
          }
        }
      }
    }
  }
  "Calib Coeff" <- w21
  "Analysis Info cluster  Out" <- w5
